vi "Aging Control Panel.vi"() -> ()   [LabVIEW 2020]
uses:
  typedefs/LED Controller Messages.ctl
  typedefs/TEC Queue Messages.ctl
  <vilib>/Utility/file.llb/Read Delimited Spreadsheet (string).vi
  Aging Control Panel_WT-v2 Backup/EC-Lab Development Package/Examples/Labview/V12/StartStopPause.vi
  Aging Control Panel_WT-v2 Backup/EC-Lab Development Package/Examples/Labview/V12/IntensityTemperature.vi
  <vilib>/Utility/file.llb/Write Delimited Spreadsheet (DBL).vi
panel:
  out "ControlTable2":dbl[][](array[numeric])
  out "Automatic Control Active H2":bool
  out "started last 2":timestamp
  out "TempArray":dbl[](array[numeric])=[29.1702938079834, 29.312671661376953, 29.52701187133789, 29.476533889770508, 31.52231216430664, 31.57969856262207, 31.603687286376953, 31.590633392333984]
  out "ControlTable1":dbl[][](array[numeric])
  out "started last":timestamp
  out "stopped":bool=TRUE
  out "Automatic Control Active H1":bool
  out "COM Done":bool
  out "Auto Done":bool
  out "TEC Done":bool
  out "index":i32
  in  "Tab Control":T1(tab)=enum."MagicControl"
  in  "ALL TEC SET A":bool caption="Light Off A"
  in  "cell A set":dbl=25.0
  in  "ALL TEC OFF B":bool caption="Light Off A"
  in  "ALL TEC ON B":bool caption="Light Off A"
  in  "ALL TEC OFF A":bool caption="Light Off A"
  in  "ALL TEC ON A":bool caption="Light Off A"
  in  "cell 1A set":dbl=25.0
  in  "cell 2A set":dbl=25.0
  in  "cell 3A set":dbl=25.0
  in  "cell 4A set":dbl=25.0
  out "cell 4A actual":dbl=29.476533889770508
  out "cell 3A actual":dbl=29.52701187133789
  out "cell 2A actual":dbl=29.312671661376953
  out "cell 1A actual":dbl=29.1702938079834
  out "Light Level B":dbl=-0.001053811659192825 caption="Light Level" format="%#_3g"
  out "Light Level A":dbl=-0.0009170305676855891 caption="Light Level" format="%#_3g"
  in  "cell 1B set":dbl=25.0
  in  "cell 2B set":dbl=25.0
  in  "cell 3B set":dbl=25.0
  in  "cell 4B set":dbl=25.0
  out "cell 4B actual":dbl=31.590633392333984
  out "cell 3B actual":dbl=31.603687286376953
  out "cell 2B actual":dbl=31.57969856262207
  out "cell 1B actual":dbl=31.52231216430664
  in  "Light Level set A":dbl(slide)=-1.0 scale=1e-05..10.0
  in  "Light Off A":bool
  in  "Light 1sun A":bool caption="Light Off A"
  in  "Light 0.1sun A":bool caption="Light Off A"
  in  "Light 0.01sun A":bool caption="Light Off A"
  in  "Light 1e-3sun A":bool caption="Light Off A"
  in  "Light 1e-4sun A":bool caption="Light Off A"
  in  "cell 1A ena":bool caption="enable"
  in  "cell 2A ena":bool caption="enable"
  in  "cell 3A ena":bool caption="enable"
  in  "cell 4A ena":bool caption="enable"
  in  "cell 1B ena":bool caption="enable"
  in  "cell 2B ena":bool caption="enable"
  in  "cell 3B ena":bool caption="enable"
  in  "cell 4B ena":bool caption="enable"
  out "TEC 1A Status":bool
  out "TEC 4A Status":bool
  out "TEC 3A Status":bool
  out "TEC 2A Status":bool
  out "TEC 4B Status":bool
  out "TEC 1B Status":bool
  out "TEC 3B Status":bool
  out "TEC 2B Status":bool
  in  "Light Level set B":dbl(slide)=-1.0 scale=1e-05..10.0
  in  "Light 1e-4sun B":bool caption="Light Off A"
  in  "Light 1e-3sun B":bool caption="Light Off A"
  in  "Light 0.01sun B":bool caption="Light Off A"
  in  "Light 0.1sun B":bool caption="Light Off A"
  in  "Light 1sun B":bool caption="Light Off A"
  in  "Light Off B":bool caption="Light Off A"
  in  "cell B set":dbl=25.0
  in  "ALL TEC SET B":bool caption="Light Off A"
  in  "Light Range A":bool=TRUE
  in  "Light Range B":bool=TRUE
  out "Temperature Monitor B":dbl[][](graph)=[[31.52231216430664, 31.57969856262207, 31.603687286376953, 31.590633392333984]]
  out "Temperature Monitor A":dbl[][](graph)=[[29.1702938079834, 29.312671661376953, 29.52701187133789, 29.476533889770508]]
  out "Light Level Monitor A":dbl(graph)=-0.0009170305676855891 caption="Cell A"
  out "Light Level Monitor B":dbl(graph)=-0.001053811659192825 caption="Cell B"
  in  "LED Auto-Connect":bool caption="Auto-Connect"
  in  "LED Disconnect":bool
  in  "LED Connect":bool
  in  "Dynamic Offset Cor.":bool=TRUE
  in  "TEC Reset":bool[](array[boolean])=[FALSE, FALSE, FALSE, FALSE, FALSE, FALSE, FALSE, FALSE] caption="Reset"
  in  "Regulation Mode A":bool=TRUE
  in  "LED Controller COM Port":refnum<visa-resource-name>="COM3"
  out "LED Controller Status":bool caption="Status"
  in  "High Light 1 Sun Level A":dbl=458.0 caption="1 Sun Level"
  in  "Low Light 1 Sun Level A":dbl=45800.0 caption="Low Light"
  in  "Light level raw A":dbl=-457.42
  in  "TEC COM Ports":refnum<visa-resource-name>[](array[refnum])=["COM6", "COM11", "COM10", "COM9", "COM4", "COM8", "COM5", "COM7"]
  out "TEC COM Status":bool[](array[boolean]) caption="Status"
  in  "TEC Auto-Detect":bool
  in  "TEC Connect":bool
  in  "TEC Disconnect":bool
  in  "TEC Address":u16(ring)=8 items=["ALL", "TEC 1A", "TEC 2A", "TEC 3A", "TEC 4A", "TEC 1B", "TEC 2B", "TEC 3B", "TEC 4B"]
  out "Diode Raw A":dbl=-1.0 format="%#_4g"
  out "Diode Raw B":dbl=-0.1 format="%#_4g"
  in  "Light level raw B":dbl=-445.97
  in  "Low Light 1 Sun Level B":dbl=44600.0 caption="Low Light"
  in  "High Light 1 Sun Level B":dbl=446.0 caption="High Light"
  in  "Regulation Mode B":bool
  out "TEC Voltage":dbl[](array[numeric])=[0.011975087225437164, 0.014526362530887127, 0.01483153272420168, 0.016552748158574104, 0.019128425046801567, 0.013830574229359627, 0.012988276779651642, 0.016076650470495224] caption="Voltage" format="%#.4g"
  out "TEC Current":dbl[](array[numeric])=[-0.0009887698106467724, -0.0016967777628451586, -0.0005615238915197551, -0.004669190384447575, -0.004687500651925802, -0.0027221685741096735, -0.0019592291209846735, -0.004602051340043545] caption="Current" format="%#.4g"
  in  "High Light Offset A":dbl=-0.5800000000000002 caption="Offset"
  in  "Low Light Offset A":dbl=-0.5100000000000001 caption="Low Light"
  in  "High Light Offset B":dbl=-0.03 caption="Offset"
  in  "Low Light Offset B":dbl=0.11999999999999998
  out "LED Driver Ground Offset (mV)":dbl=0.4
  in  "TEC Auto-Connect":bool caption="Auto-Connect"
  in  "TEC monitor\nperiod (ms)":i32=500
  in  "LED monitor\nperiod (ms)":i32=500
  in  "LED Slide reactivity (ms)":i32=250
  in  "TimingList2":i32(listbox)=-1
  out "Active Row 2":i32 caption="Active Row"
  out "started at 2":timestamp caption="started at"
  in  "RemoveRow1":bool caption="Light Off A"
  in  "AddRow1":bool caption="Light Off A"
  in  "SaveControlTable":bool caption="Light Off A"
  in  "LoadControlTable":bool caption="Light Off A"
  in  "TimingList1":i32(listbox)=-1
  in  "StartMagicControl":bool caption="Light Off A"
  in  "StopMagicControl":bool caption="Light Off A"
  out "started at":timestamp
  out "ElapsedTime":dbl
  out "Active Row":i32
  out "Current Row":dbl
  in  "loop to row":i32
  in  "loop to row 2":i32 caption="loop to row"
  out "Current Row 2":dbl caption="Current Row"
  out "ElapsedTime 2":dbl caption="ElapsedTime"
  in  "LoadControlTable 2":bool caption="Light Off A"
  in  "SaveControlTable 2":bool caption="Light Off A"
  in  "AddRow2":bool caption="Light Off A"
  in  "RemoveRow2":bool caption="Light Off A"
  in  "StartMagicControl 2":bool caption="Light Off A"
  in  "StopMagicControl 2":bool caption="Light Off A"
  out "StartStopPauseArray1":bool[][](array[boolean]) caption="Holder 1\nStart Stop Pause"
  out "StartStopPauseArray2":bool[][](array[boolean]) caption="Holder 2\nStart Stop Pause"
  in  "stop":bool
  # "3A"
  # "4B"
  # "3B"
  # "4A"
  # "1B"
  # "2A"
  # "1A"
  # "2B"
  # "LED A"
  # "LED B"
  # "1 Sun Level"
  # "High Light"
  # "Active (light green, on) entries will overwrite the commands in the AgingControl.\nNon-active entries will not do anything."
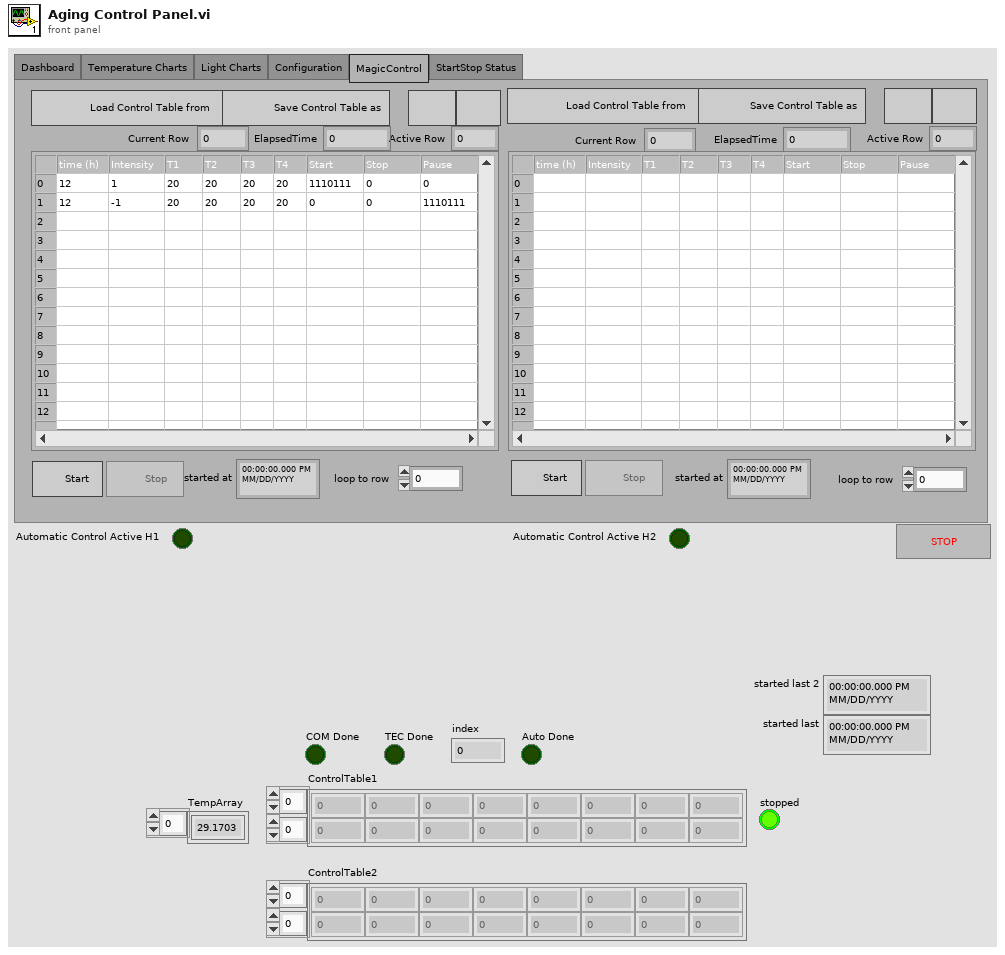
[diagram p1: front panel]
types:
  T1 = enum32{"Dashboard", "Temperature Charts", "Light Charts", "Configuration", "MagicControl", "StartStop Status"}
  T2 = cluster{"A Current":bool, "B Current":bool, "A lastupdate":u32, "B lastupdate":u32, "SetRange A":bool, "SetRange B":bool}
  T3 = cluster{"MODE A":bool, "MODE B":bool, "RANGE A":bool, "RANGE B":bool}
  T4 = typedef "TEC Queue Messages.ctl" = enum16{"Auto Detect", "Connect", "Disconnect", "Exit", "Set Temp", "Output Ena", "RESET"}
  T5 = typedef "LED Controller Messages.ctl" = enum16{"Connect", "Disconnect", "Exit", "Set Mode A", "Set Mode B", "Set Range A", "Set Range B", "Set Output A", "Set Output B"}
  T6 = enum8{"Enabled", "Disabled", "Disabled and Grayed Out"}
  T7 = cluster{"LED Controller COM Port":refnum<visa-resource-name>, i32}
  T8 = cluster{"LED Controller COM Port":refnum<visa-resource-name>, "TEC ID":i32}
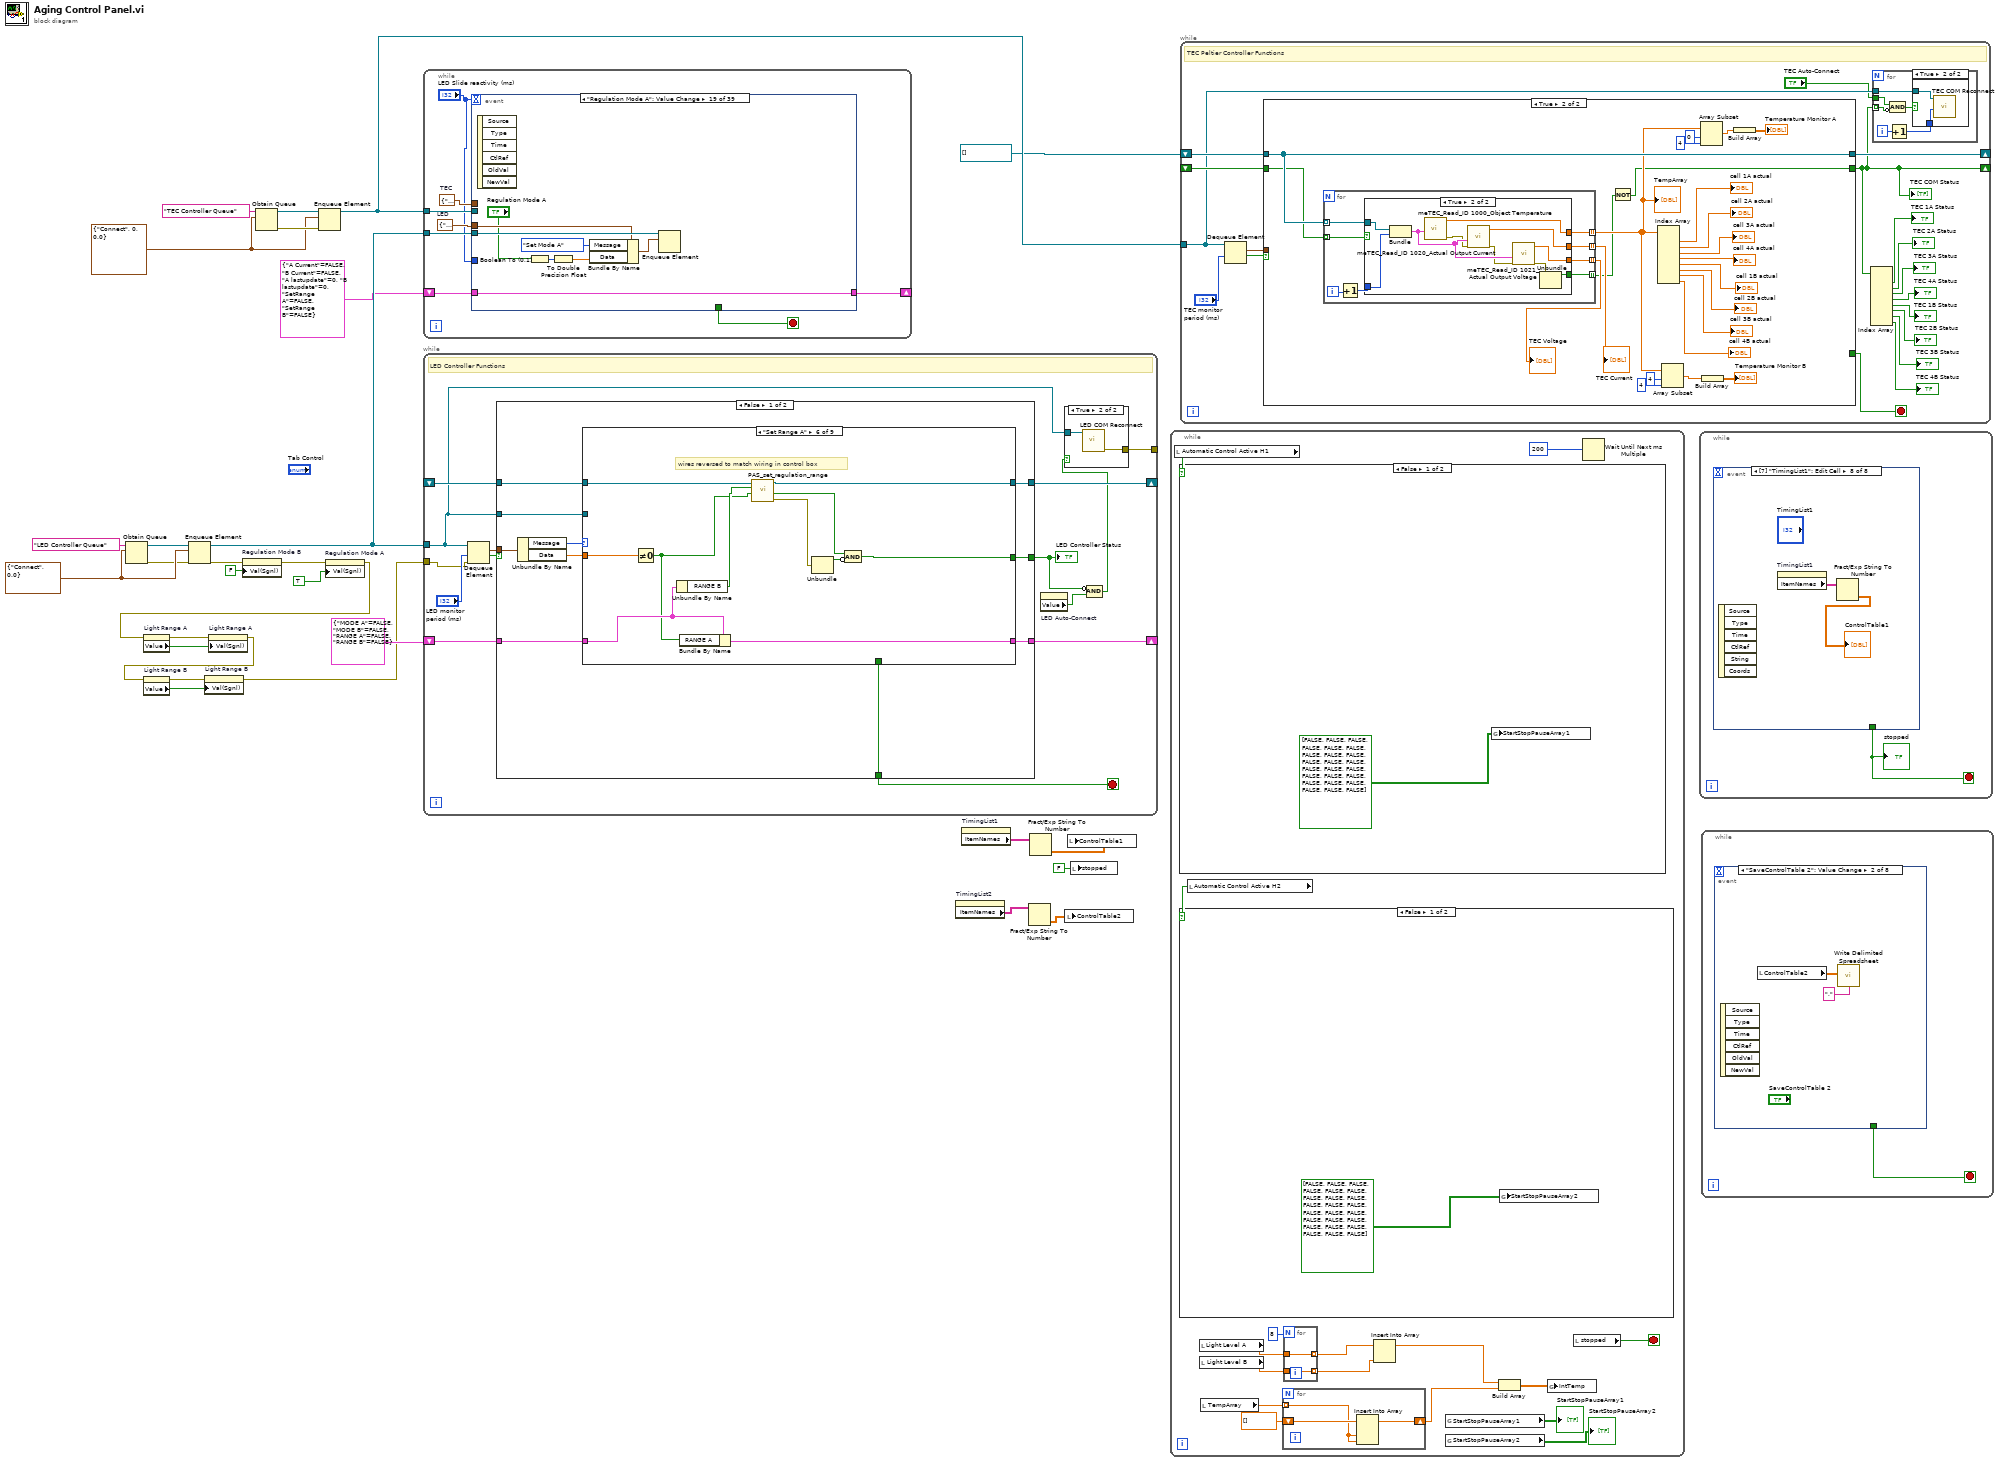
[diagram p0: block diagram]
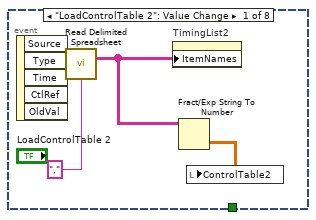
[diagram p2: hidden frame]
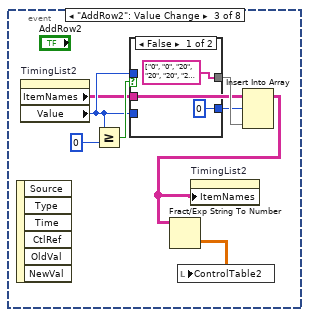
[diagram p3: hidden frame]
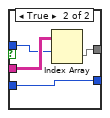
[diagram p4: hidden frame]
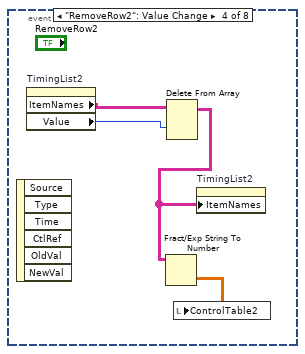
[diagram p5: hidden frame]
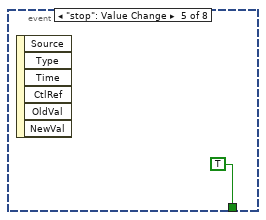
[diagram p6: hidden frame]
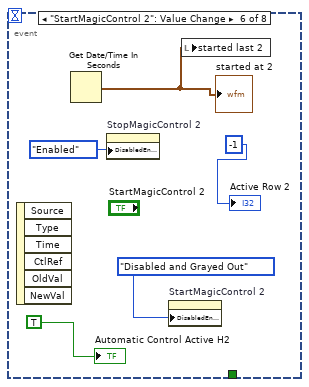
[diagram p7: hidden frame]
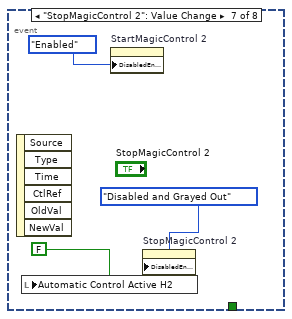
[diagram p8: hidden frame]
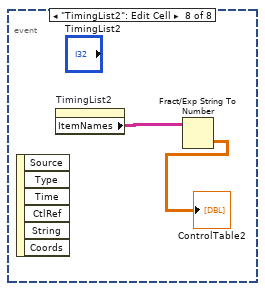
[diagram p9: hidden frame]
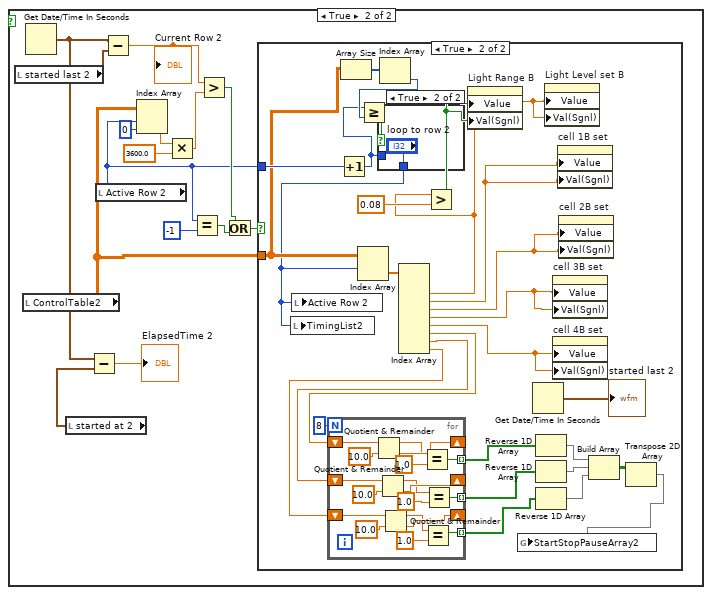
[diagram p10: hidden frame]
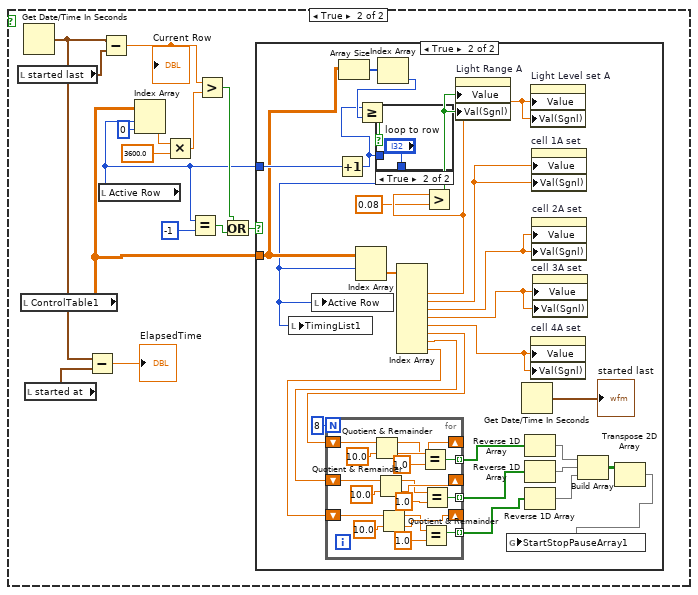
[diagram p13: hidden frame]
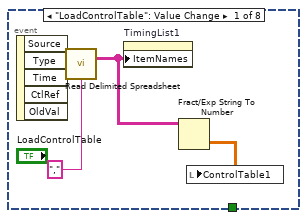
[diagram p16: hidden frame]
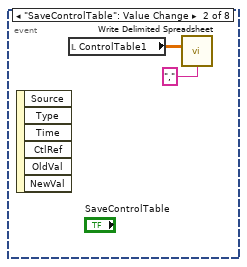
[diagram p17: hidden frame]
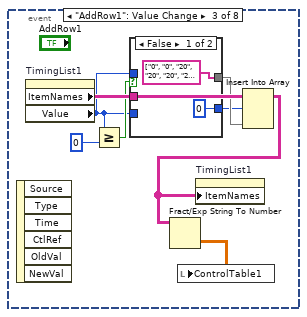
[diagram p18: hidden frame]
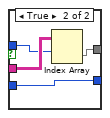
[diagram p19: hidden frame]
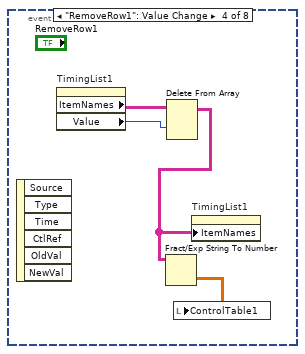
[diagram p20: hidden frame]
diagram:
  w24 = cluster{"Message":T4, "TEC ID":i32, "Data":dbl} {"Message"=enum."Connect", "TEC ID"=0, "Data"=0.0}
  w27 = cluster{"Message":T5, "Data":dbl} {"Message"=enum."Connect", "Data"=0.0}
  n1 = Obtain Queue(name (unnamed)="LED Controller Queue", element data type=w27) -> (queue out=w28:refnum<queue>, error out=w26:errorcluster)  [unwired: 3 in, 1 out]
  n2 = Enqueue Element(queue=w28, element=w27, error in (no error)=w26) -> (queue out=w17:refnum<queue>, error out=w18:errorcluster)  [unwired: 1 in, 1 out]
  n3 = property on="Regulation Mode B" class="Bool (strict)"(error in=w18, "Val(Sgnl)"=FALSE ("Value (Signaling)")) -> (error out=w16:errorcluster)  [unwired: 1 in, 1 out]
  n4 = Obtain Queue(name (unnamed)="TEC Controller Queue", element data type=w24) -> (queue out=w23:refnum<queue>, error out=w25:errorcluster)  [unwired: 3 in, 1 out]
  n5 = Enqueue Element(queue=w23, element=w24, error in (no error)=w25) -> (queue out=w21:refnum<queue>)  [unwired: 1 in, 2 out]
  n6 = property on="Regulation Mode A" class="Bool (strict)"(error in=w16, "Val(Sgnl)"=TRUE ("Value (Signaling)")) -> (error out=w9:errorcluster)  [unwired: 1 in, 1 out]
  n7 = property on="Light Range A" class="Bool (strict)"(error in=w9) -> (error out=w12:errorcluster, "Value"=w13:bool)  [unwired: 1 in, 1 out]
  n8 = property on="Light Range A" class="Bool (strict)"(error in=w12, "Val(Sgnl)"=w13) -> (error out=w8:errorcluster)  [unwired: 1 in, 1 out]
  n9 = property on="Light Range B" class="Bool (strict)"(error in=w8) -> (error out=w10:errorcluster, "Value"=w11:bool)  [unwired: 1 in, 1 out]
  n10 = property on="Light Range B" class="Bool (strict)"(error in=w10, "Val(Sgnl)"=w11) -> (error out=w7:errorcluster)  [unwired: 1 in, 1 out]
  n11 = while {
    tunnel: w17 -> [w36]
    tunnel: w21 -> [w34]
    shift-right: [w31] -> _
    shift-left: T2 {"A Current"=FALSE, "B Current"=FALSE, "A lastupdate"=0, "B lastupdate"=0, "SetRange A"=FALSE, "SetRange B"=FALSE} -> [w32]
    stop <- w37 stop-if-true
    w33 = cluster{"Message":T4, "TEC ID":i32, "Data":dbl} {"Message"=enum."Connect", "TEC ID"=0, "Data"=0.0}  # TEC
    w35 = cluster{"Message":T5, "Data":dbl} {"Message"=enum."Set Output B", "Data"=0.0}  # LED
    n12 = event shown="[18] \"Regulation Mode A\": Value Change" {
      selector: _ -> [_ _ _ _ _ _ _ _ _ _ _ _ _ _ _ _ _ _ _ _ _ _ _ _ _ _ _ _ _ _ _ _ _ _ _ _ _ _ _]
      dyn-events: _ -> [_ _ _ _ _ _ _ _ _ _ _ _ _ _ _ _ _ _ _ _ _ _ _ _ _ _ _ _ _ _ _ _ _ _ _ _ _ _ _]
      timeout: "LED Slide reactivity (ms)" -> [_ _ _ _ _ _ _ _ _ _ _ _ _ _ _ _ _ _ _ _ _ _ _ _ _ _ _ _ _ _ _ _ _ _ _ _ _ _ _]
      tunnel: [_ TRUE _ _ _ _ _ _ _ _ _ _ _ _ _ _ _ _ _ _ _ _ _ _ _ _ _ _ _ _ _ _ _ _ _ _ _ _ _] -> w37
      tunnel: w36 -> [_ w66 _ _ _ _ _ _ _ _ _ _ _ _ _ _ w152 w170 w191 w199 w207 w236 _ _ _ _ _ _ _ _ _ _ _ _ _ w379 w386 _ w428]
      tunnel: w35 -> [_ w58 _ _ _ _ _ _ _ _ _ _ _ _ _ _ w151 w169 w190 w198 w204 w233 _ _ _ _ _ _ _ _ _ _ _ _ _ w381 w385 _ w430]
      tunnel: w34 -> [_ w69 _ _ _ _ _ _ _ _ _ _ _ _ _ _ _ _ _ _ _ _ w264 w277 _ _ _ _ _ _ w326 _ w357 w366 w375 _ _ w407 _]
      tunnel: w33 -> [_ w64 _ _ _ _ _ _ _ _ _ _ _ _ _ _ _ _ _ _ _ _ w263 w276 _ _ _ _ _ _ w325 _ w356 w365 w374 _ _ w406 _]
      tunnel: w32 -> [w42 w56 w75 w101 w124 w126 w128 w130 w132 w134 w136 w138 w140 w142 w144 w146 w149 w168 w184 w192 w202 w231 w256 w266 w278 w286 w294 w302 w310 w315 w320 w329 w350 w358 w367 w376 w384 w405 w425]
      tunnel: [w38 w56 w74 w99 w124 w126 w128 w130 w132 w134 w136 w138 w140 w142 w144 w146 w148 w167 w184 w192 w201 w230 w256 w266 w278 w286 w294 w302 w310 w315 w320 w329 w350 w358 w367 w376 w384 w405 w425] -> w31
      tunnel: "LED Slide reactivity (ms)" -> [_ _ w72 w98 _ _ _ _ _ _ _ _ _ _ _ _ _ _ _ _ _ _ _ _ _ _ _ _ _ _ _ _ _ _ _ _ _ _ _]
      event Timeout {
        n13 = event-data() -> ("Time"=w40:u32)  [unwired: 1 in, 2 out]
        n14 = Unbundle By Name(w42) -> ("A Current"=w43:bool, "B Current"=w39:bool)
        n15 = case shown="False" w43 {
          tunnel: w42 -> [w53 w55]
          tunnel: w40 -> [w52 _]
          tunnel: [w50 w55] -> w41
          frame False {
            n16 = property on="Light level raw A" class="DigNum (strict)"() -> ("Value"=w54:dbl)  [unwired: 2 in, 2 out]
            n17 = Bundle By Name(cluster=w53, "A Current"=TRUE, "A lastupdate"=w52) -> (w50:T2)
            n18 = property on="Light level raw A" class="DigNum (strict)"("Val(Sgnl)"=w54) -> ()  [unwired: 2 in, 2 out]
          }
          frame True {
          }
        }
        n19 = case shown="False" w39 {
          tunnel: w41 -> [w47 w49]
          tunnel: w40 -> [w46 _]
          tunnel: [w44 w49] -> w38
          frame False {
            n20 = property on="Light level raw B" class="DigNum (strict)"() -> ("Value"=w48:dbl)  [unwired: 2 in, 2 out]
            n21 = Bundle By Name(cluster=w47, "B Current"=TRUE ("A Current"), "B lastupdate"=w46) -> (w44:T2)
            n22 = property on="Light level raw B" class="DigNum (strict)"("Val(Sgnl)"=w48) -> ()  [unwired: 2 in, 2 out]
          }
          frame True {
          }
        }
      }
      event "stop": Value Change {
        n23 = event-data() -> ()  [unwired: 1 in, 6 out]
        n24 = Bundle By Name(cluster=w58, "Message"=LED_Controller_Messages."Disconnect") -> (w59:cluster{"Message":T5, "Data":dbl})
        n25 = Bundle By Name(cluster=w58, "Message"=LED_Controller_Messages."Exit") -> (w57:cluster{"Message":T5, "Data":dbl})
        n26 = Bundle By Name(cluster=w64, "Message"=TEC_Queue_Messages."Disconnect") -> (w67:cluster{"Message":T4, "TEC ID":i32, "Data":dbl})
        n27 = Bundle By Name(cluster=w64, "Message"=TEC_Queue_Messages."Exit") -> (w62:cluster{"Message":T4, "TEC ID":i32, "Data":dbl})
        n28 = Enqueue Element(queue=w66, element=w59) -> (queue out=w61:refnum<queue>)  [unwired: 2 in, 2 out]
        n29 = Enqueue Element(queue=w69, element=w67) -> (queue out=w63:refnum<queue>)  [unwired: 2 in, 2 out]
        n30 = Enqueue Element(queue=w61, element=w57) -> ()  [unwired: 2 in, 3 out]
        n31 = Enqueue Element(queue=w63, element=w62) -> ()  [unwired: 2 in, 3 out]
      }
      event "Light Level set B": Value Change {
        n32 = event-data() -> ("Time"=w73:u32)  [unwired: 1 in, 5 out]
        n33 = Unbundle By Name(w75) -> ("B lastupdate"=w78:u32)
        n34 = property on="Light Range B" class="Bool (strict)"() -> ("Value"=w82:bool)  [unwired: 2 in, 2 out]
        n35 = Subtract(x=w73, y=w78) -> (x-y=w77:u32)
        n36 = Select(t="High Light 1 Sun Level B", s=w82, f="Low Light 1 Sun Level B") -> (s? t:f=w87:dbl)
        n37 = Greater?(x=w77, y=w72) -> (0:w76:bool)
        n38 = Multiply(x=w87, y="Light Level set B") -> (x*y=w81:dbl)
        n39 = Select(t="High Light Offset B", s=w82, f="Low Light Offset B") -> (s? t:f=w79:dbl)
        n40 = Subtract(x=w81, y=w79) -> (x-y=w80:dbl)
        n41 = case shown="True" w76 {
          selector: w76 -> [w90 w93]
          tunnel: w80 -> [w89 w97]
          tunnel: w75 -> [w92 w96]
          tunnel: [w91 w95] -> w74
          tunnel: w73 -> [_ w94]
          frame False {
            n42 = Bundle By Name(cluster=w92, "B Current"=w90) -> (w91:T2)
            n43 = property on="Light level raw B" class="DigNum (strict)"("Value"=w89) -> ()  [unwired: 2 in, 2 out]
          }
          frame True {
            n44 = Bundle By Name(cluster=w96, "B Current"=w93, "B lastupdate"=w94) -> (w95:T2)
            n45 = property on="Light level raw B" class="DigNum (strict)"("Val(Sgnl)"=w97) -> ()  [unwired: 2 in, 2 out]
          }
        }
      }
      event "Light Level set A": Value Change {
        n46 = event-data() -> ("Time"=w100:u32)  [unwired: 1 in, 5 out]
        n47 = Unbundle By Name(w101) -> ("A lastupdate"=w104:u32)
        n48 = property on="Light Range A" class="Bool (strict)"() -> ("Value"=w108:bool)  [unwired: 2 in, 2 out]
        n49 = Subtract(x=w100, y=w104) -> (x-y=w103:u32)
        n50 = Select(t="High Light 1 Sun Level A", s=w108, f="Low Light 1 Sun Level A") -> (s? t:f=w113:dbl)
        n51 = Greater?(x=w103, y=w98) -> (0:w102:bool)
        n52 = Multiply(x=w113, y="Light Level set A") -> (x*y=w107:dbl)
        n53 = Select(t="High Light Offset A", s=w108, f="Low Light Offset A") -> (s? t:f=w105:dbl)
        n54 = Subtract(x=w107, y=w105) -> (x-y=w106:dbl)
        n55 = case shown="False" w102 {
          selector: w102 -> [w117 w121]
          tunnel: w106 -> [w115 w123]
          tunnel: w101 -> [w118 w122]
          tunnel: w100 -> [_ w120]
          tunnel: [w116 w119] -> w99
          frame False {
            n56 = Bundle By Name(cluster=w118, "A Current"=w117) -> (w116:T2)
            n57 = property on="Light level raw A" class="DigNum (strict)"("Value"=w115) -> ()  [unwired: 2 in, 2 out]
          }
          frame True {
            n58 = Bundle By Name(cluster=w122, "A Current"=w121, "A lastupdate"=w120) -> (w119:T2)
            n59 = property on="Light level raw A" class="DigNum (strict)"("Val(Sgnl)"=w123) -> ()  [unwired: 2 in, 2 out]
          }
        }
      }
      event "Light 1sun B": Value Change {
        n60 = event-data() -> ()  [unwired: 1 in, 6 out]
        n61 = property on="Light Level set B" class="Slide (strict)"("Val(Sgnl)"=1.0 ("Value (Signaling)")) -> ()  [unwired: 2 in, 2 out]
      }
      event "Light 1sun A": Value Change {
        n62 = event-data() -> ()  [unwired: 1 in, 6 out]
        n63 = property on="Light Level set A" class="Slide (strict)"("Val(Sgnl)"=1.0 ("Value (Signaling)")) -> ()  [unwired: 2 in, 2 out]
      }
      event "Light 0.1sun B": Value Change {
        n64 = event-data() -> ()  [unwired: 1 in, 6 out]
        n65 = property on="Light Level set B" class="Slide (strict)"("Val(Sgnl)"=0.1 ("Value (Signaling)")) -> ()  [unwired: 2 in, 2 out]
      }
      event "Light 0.1sun A": Value Change {
        n66 = event-data() -> ()  [unwired: 1 in, 6 out]
        n67 = property on="Light Level set A" class="Slide (strict)"("Val(Sgnl)"=0.1 ("Value (Signaling)")) -> ()  [unwired: 2 in, 2 out]
      }
      event "Light 0.01sun B": Value Change {
        n68 = event-data() -> ()  [unwired: 1 in, 6 out]
        n69 = property on="Light Level set B" class="Slide (strict)"("Val(Sgnl)"=0.01 ("Value (Signaling)")) -> ()  [unwired: 2 in, 2 out]
      }
      event "Light 0.01sun A": Value Change {
        n70 = event-data() -> ()  [unwired: 1 in, 6 out]
        n71 = property on="Light Level set A" class="Slide (strict)"("Val(Sgnl)"=0.01 ("Value (Signaling)")) -> ()  [unwired: 2 in, 2 out]
      }
      event "Light 1e-3sun B": Value Change {
        n72 = event-data() -> ()  [unwired: 1 in, 6 out]
        n73 = property on="Light Level set B" class="Slide (strict)"("Val(Sgnl)"=0.001 ("Value (Signaling)")) -> ()  [unwired: 2 in, 2 out]
      }
      event "Light 1e-3sun A": Value Change {
        n74 = event-data() -> ()  [unwired: 1 in, 6 out]
        n75 = property on="Light Level set A" class="Slide (strict)"("Val(Sgnl)"=0.001 ("Value (Signaling)")) -> ()  [unwired: 2 in, 2 out]
      }
      event "Light 1e-4sun B": Value Change {
        n76 = event-data() -> ()  [unwired: 1 in, 6 out]
        n77 = property on="Light Level set B" class="Slide (strict)"("Val(Sgnl)"=0.0001 ("Value (Signaling)")) -> ()  [unwired: 2 in, 2 out]
      }
      event "Light 1e-4sun A": Value Change {
        n78 = event-data() -> ()  [unwired: 1 in, 6 out]
        n79 = property on="Light Level set A" class="Slide (strict)"("Val(Sgnl)"=0.0001 ("Value (Signaling)")) -> ()  [unwired: 2 in, 2 out]
      }
      event "Light Off B": Value Change {
        n80 = event-data() -> ()  [unwired: 1 in, 6 out]
        n81 = property on="Light Level set B" class="Slide (strict)"("Val(Sgnl)"=-1.0 ("Value (Signaling)")) -> ()  [unwired: 2 in, 2 out]
      }
      event "Light Off A": Value Change {
        n82 = event-data() -> ()  [unwired: 1 in, 6 out]
        n83 = property on="Light Level set A" class="Slide (strict)"("Val(Sgnl)"=-1.0 ("Value (Signaling)")) -> ()  [unwired: 2 in, 2 out]
      }
      event "Light Range B": Value Change {
        n84 = event-data() -> ()  [unwired: 1 in, 6 out]
        n85 = property on="Light Level set B" class="Slide (strict)"() -> (error out=w153:errorcluster, "Value"=w154:dbl)  [unwired: 2 in, 1 out]
        n86 = case shown="False" "Light Range B" {
          selector: "Light Range B" -> [w156 _]
          tunnel: w152 -> [w162 _]
          tunnel: w151 -> [w161 _]
          tunnel: w149 -> [w155 w165]
          tunnel: [w155 w164] -> w148
          frame False {
            n87 = Boolean To (0,1)(Boolean=w156) -> (0, 1=w159:i16)
            n88 = To Double Precision Float(number=w159) -> (double precision float=w158:dbl)
            n89 = Bundle By Name(cluster=w161, "Message"=LED_Controller_Messages."Set Range B", "Data"=w158) -> (w157:cluster{"Message":T5, "Data":dbl})
            n90 = Enqueue Element(queue=w162, element=w157) -> ()  [unwired: 2 in, 3 out]
          }
          frame True {
            n91 = Bundle By Name(cluster=w165, "SetRange B"=TRUE) -> (w164:T2)
          }
        }
        n92 = property on="Light Level set B" class="Slide (strict)"(error in=w153, "Val(Sgnl)"=w154) -> ()  [unwired: 1 in, 2 out]
      }
      event "Light Range A": Value Change {
        n93 = event-data() -> ()  [unwired: 1 in, 6 out]
        n94 = property on="Light Level set A" class="Slide (strict)"() -> (error out=w171:errorcluster, "Value"=w172:dbl)  [unwired: 2 in, 1 out]
        n95 = case shown="True" "Light Range A" {
          selector: "Light Range A" -> [w174 _]
          tunnel: w170 -> [w180 _]
          tunnel: w169 -> [w179 _]
          tunnel: w168 -> [w173 w183]
          tunnel: [w173 w182] -> w167
          frame False {
            n96 = Boolean To (0,1)(Boolean=w174) -> (0, 1=w177:i16)
            n97 = To Double Precision Float(number=w177) -> (double precision float=w176:dbl)
            n98 = Bundle By Name(cluster=w179, "Message"=LED_Controller_Messages."Set Range A", "Data"=w176) -> (w175:cluster{"Message":T5, "Data":dbl})
            n99 = Enqueue Element(queue=w180, element=w175) -> ()  [unwired: 2 in, 3 out]
          }
          frame True {
            n100 = Bundle By Name(cluster=w183, "SetRange A"=TRUE ("SetRange B")) -> (w182:T2)
          }
        }
        n101 = property on="Light Level set A" class="Slide (strict)"(error in=w171, "Val(Sgnl)"=w172) -> ()  [unwired: 1 in, 2 out]
      }
      event "Regulation Mode A": Value Change {
        n102 = event-data() -> ()  [unwired: 1 in, 6 out]
        n103 = Boolean To (0,1)(Boolean="Regulation Mode A") -> (0, 1=w188:i16)
        n104 = To Double Precision Float(number=w188) -> (double precision float=w187:dbl)
        n105 = Bundle By Name(cluster=w190, "Message"=LED_Controller_Messages."Set Mode A", "Data"=w187) -> (w186:cluster{"Message":T5, "Data":dbl})
        n106 = Enqueue Element(queue=w191, element=w186) -> ()  [unwired: 2 in, 3 out]
      }
      event "Regulation Mode B": Value Change {
        n107 = event-data() -> ()  [unwired: 1 in, 6 out]
        n108 = Boolean To (0,1)(Boolean="Regulation Mode B") -> (0, 1=w196:i16)
        n109 = To Double Precision Float(number=w196) -> (double precision float=w195:dbl)
        n110 = Bundle By Name(cluster=w198, "Message"=LED_Controller_Messages."Set Mode B", "Data"=w195) -> (w194:cluster{"Message":T5, "Data":dbl})
        n111 = Enqueue Element(queue=w199, element=w194) -> ()  [unwired: 2 in, 3 out]
      }
      event "Light level raw B": Value Change {
        n112 = event-data() -> ()  [unwired: 1 in, 6 out]
        n113 = Unbundle By Name(w202) -> ("SetRange B"=w203:bool)
        n114 = In Range and Coerce(upper limit=4900.0, x="Light level raw B", lower limit=-3.0) -> (coerced(x)=w206:dbl)  [unwired: 1 out]
        n115 = Bundle By Name(cluster=w204, "Message"=LED_Controller_Messages."Set Output B", "Data"=w206) -> (w211:cluster{"Message":T5, "Data":dbl})
        n116 = Enqueue Element(queue=w207, element=w211) -> (queue out=w205:refnum<queue>, error out=w200:errorcluster)  [unwired: 2 in, 1 out]
        n117 = case shown="True" w203 {
          selector: w203 -> [_ w216]
          tunnel: w205 -> [_ w225]
          tunnel: w204 -> [_ w224]
          tunnel: w202 -> [w213 w219]
          tunnel: [w213 w217] -> w201
          tunnel: w200 -> [_ w215]
          frame False {
          }
          frame True {
            n118 = flat-sequence {
              tunnel: w215 -> [w226]
              tunnel: [w226] -> w214
              frame #0 {
                n119 = Wait (ms)(milliseconds to wait=u32 100) -> ()  [unwired: 1 out]
              }
            }
            n120 = Boolean To (0,1)(Boolean=w216) -> (0, 1=w222:i16)
            n121 = Bundle By Name(cluster=w219, "SetRange B"=FALSE) -> (w217:T2)
            n122 = To Double Precision Float(number=w222) -> (double precision float=w221:dbl)
            n123 = Bundle By Name(cluster=w224, "Message"=LED_Controller_Messages."Set Range B", "Data"=w221) -> (w220:cluster{"Message":T5, "Data":dbl})
            n124 = Enqueue Element(queue=w225, element=w220, error in (no error)=w214) -> ()  [unwired: 1 in, 3 out]
          }
        }
      }
      event "Light level raw A": Value Change {
        n125 = event-data() -> ()  [unwired: 1 in, 6 out]
        n126 = Unbundle By Name(w231) -> ("SetRange A"=w232:bool)
        n127 = In Range and Coerce(upper limit=4900.0, x="Light level raw A", lower limit=-3.0) -> (coerced(x)=w235:dbl)  [unwired: 1 out]
        n128 = Bundle By Name(cluster=w233, "Message"=LED_Controller_Messages."Set Output A", "Data"=w235) -> (w239:cluster{"Message":T5, "Data":dbl})
        n129 = Enqueue Element(queue=w236, element=w239) -> (queue out=w234:refnum<queue>, error out=w229:errorcluster)  [unwired: 2 in, 1 out]
        n130 = case shown="True" w232 {
          selector: w232 -> [_ w244]
          tunnel: w234 -> [_ w253]
          tunnel: w233 -> [_ w252]
          tunnel: w231 -> [w241 w247]
          tunnel: [w241 w245] -> w230
          tunnel: w229 -> [_ w243]
          frame False {
          }
          frame True {
            n131 = flat-sequence {
              tunnel: w243 -> [w254]
              tunnel: [w254] -> w242
              frame #0 {
                n132 = Wait (ms)(milliseconds to wait=u32 100) -> ()  [unwired: 1 out]
              }
            }
            n133 = Boolean To (0,1)(Boolean=w244) -> (0, 1=w250:i16)
            n134 = Bundle By Name(cluster=w247, "SetRange A"=FALSE ("SetRange B")) -> (w245:T2)
            n135 = To Double Precision Float(number=w250) -> (double precision float=w249:dbl)
            n136 = Bundle By Name(cluster=w252, "Message"=LED_Controller_Messages."Set Range A", "Data"=w249) -> (w248:cluster{"Message":T5, "Data":dbl})
            n137 = Enqueue Element(queue=w253, element=w248, error in (no error)=w242) -> ()  [unwired: 1 in, 3 out]
          }
        }
      }
      event "cell 1A set", "cell 2A set", "cell 3A set", "cell 4A set", "cell 1B set", "cell 2B set", "cell 3B set", "cell 4B set": Value Change {
        n138 = event-data() -> ("CtlRef"=w265:refnum<vi>, "NewVal"=w260:dbl)  [unwired: 1 in, 4 out]
        n139 = To More Generic Class(target class=refnum<vi> refnum ("reference"), reference=w265) -> (generic class reference=w258:refnum<vi>)
        n140 = call "Extract Control Index.vi"("reference"=w258) -> ("index"=w261:i32)  [unwired: 10 in]
        n141 = Bundle By Name(cluster=w263, "Message"=TEC_Queue_Messages."Set Temp", "TEC ID"=w261, "Data"=w260) -> (w259:cluster{"Message":T4, "TEC ID":i32, "Data":dbl})
        n142 = Enqueue Element(queue=w264, element=w259) -> ()  [unwired: 2 in, 3 out]
      }
      event "cell 1A ena", "cell 2A ena", "cell 3A ena", "cell 4A ena", "cell 1B ena", "cell 2B ena", "cell 3B ena", "cell 4B ena": Value Change {
        n143 = event-data() -> ("CtlRef"=w269:refnum<vi>, "NewVal"=w273:bool)  [unwired: 1 in, 4 out]
        n144 = To More Generic Class(target class=refnum<vi> refnum ("reference"), reference=w269) -> (generic class reference=w268:refnum<vi>)
        n145 = Boolean To (0,1)(Boolean=w273) -> (0, 1=w271:i16)
        n146 = To Double Precision Float(number=w271) -> (double precision float=w270:dbl)
        n147 = call "Extract Control Index.vi"("reference"=w268) -> ("index"=w274:i32)  [unwired: 10 in]
        n148 = Bundle By Name(cluster=w276, "Message"=TEC_Queue_Messages."Output Ena", "TEC ID"=w274, "Data"=w270) -> (w272:cluster{"Message":T4, "TEC ID":i32, "Data":dbl})
        n149 = Enqueue Element(queue=w277, element=w272) -> ()  [unwired: 2 in, 3 out]
      }
      event "ALL TEC ON A": Value Change {
        n150 = event-data() -> ()  [unwired: 1 in, 6 out]
        n151 = property on="cell 1A ena" class="Bool (strict)"("Val(Sgnl)"=TRUE ("cell 1A ena")) -> (error out=w285:errorcluster)  [unwired: 2 in, 1 out]
        n152 = property on="cell 2A ena" class="Bool (strict)"(error in=w285, "Val(Sgnl)"=TRUE ("cell 2A ena")) -> (error out=w284:errorcluster)  [unwired: 1 in, 1 out]
        n153 = property on="cell 3A ena" class="Bool (strict)"(error in=w284, "Val(Sgnl)"=TRUE ("cell 3A ena")) -> (error out=w283:errorcluster)  [unwired: 1 in, 1 out]
        n154 = property on="cell 4A ena" class="Bool (strict)"(error in=w283, "Val(Sgnl)"=TRUE ("Value (Signaling)")) -> ()  [unwired: 1 in, 2 out]
      }
      event "ALL TEC OFF A": Value Change {
        n155 = event-data() -> ()  [unwired: 1 in, 6 out]
        n156 = property on="cell 1A ena" class="Bool (strict)"("Val(Sgnl)"=FALSE ("cell 1A ena")) -> (error out=w293:errorcluster)  [unwired: 2 in, 1 out]
        n157 = property on="cell 2A ena" class="Bool (strict)"(error in=w293, "Val(Sgnl)"=FALSE ("cell 2A ena")) -> (error out=w292:errorcluster)  [unwired: 1 in, 1 out]
        n158 = property on="cell 3A ena" class="Bool (strict)"(error in=w292, "Val(Sgnl)"=FALSE ("cell 3A ena")) -> (error out=w291:errorcluster)  [unwired: 1 in, 1 out]
        n159 = property on="cell 4A ena" class="Bool (strict)"(error in=w291, "Val(Sgnl)"=FALSE ("Value (Signaling)")) -> ()  [unwired: 1 in, 2 out]
      }
      event "ALL TEC ON B": Value Change {
        n160 = event-data() -> ()  [unwired: 1 in, 6 out]
        n161 = property on="cell 1B ena" class="Bool (strict)"("Val(Sgnl)"=TRUE ("cell 1A ena")) -> (error out=w301:errorcluster)  [unwired: 2 in, 1 out]
        n162 = property on="cell 2B ena" class="Bool (strict)"(error in=w301, "Val(Sgnl)"=TRUE ("cell 2A ena")) -> (error out=w300:errorcluster)  [unwired: 1 in, 1 out]
        n163 = property on="cell 3B ena" class="Bool (strict)"(error in=w300, "Val(Sgnl)"=TRUE ("cell 3A ena")) -> (error out=w299:errorcluster)  [unwired: 1 in, 1 out]
        n164 = property on="cell 4B ena" class="Bool (strict)"(error in=w299, "Val(Sgnl)"=TRUE ("Value (Signaling)")) -> ()  [unwired: 1 in, 2 out]
      }
      event "ALL TEC OFF B": Value Change {
        n165 = event-data() -> ()  [unwired: 1 in, 6 out]
        n166 = property on="cell 1B ena" class="Bool (strict)"("Val(Sgnl)"=FALSE ("cell 1A ena")) -> (error out=w309:errorcluster)  [unwired: 2 in, 1 out]
        n167 = property on="cell 2B ena" class="Bool (strict)"(error in=w309, "Val(Sgnl)"=FALSE ("cell 2A ena")) -> (error out=w308:errorcluster)  [unwired: 1 in, 1 out]
        n168 = property on="cell 3B ena" class="Bool (strict)"(error in=w308, "Val(Sgnl)"=FALSE ("cell 3A ena")) -> (error out=w307:errorcluster)  [unwired: 1 in, 1 out]
        n169 = property on="cell 4B ena" class="Bool (strict)"(error in=w307, "Val(Sgnl)"=FALSE ("Value (Signaling)")) -> ()  [unwired: 1 in, 2 out]
      }
      event "ALL TEC SET A": Value Change {
        n170 = event-data() -> ()  [unwired: 1 in, 6 out]
        n171 = property on="cell 1A set" class="DigNum (strict)"("Val(Sgnl)"="cell A set") -> (error out=w314:errorcluster)  [unwired: 2 in, 1 out]
        n172 = property on="cell 2A set" class="DigNum (strict)"(error in=w314, "Val(Sgnl)"="cell A set") -> (error out=w313:errorcluster)  [unwired: 1 in, 1 out]
        n173 = property on="cell 3A set" class="DigNum (strict)"(error in=w313, "Val(Sgnl)"="cell A set") -> (error out=w312:errorcluster)  [unwired: 1 in, 1 out]
        n174 = property on="cell 4A set" class="DigNum (strict)"(error in=w312, "Val(Sgnl)"="cell A set") -> ()  [unwired: 1 in, 2 out]
      }
      event "ALL TEC SET B": Value Change {
        n175 = event-data() -> ()  [unwired: 1 in, 6 out]
        n176 = property on="cell 1B set" class="DigNum (strict)"("Val(Sgnl)"="cell B set") -> (error out=w319:errorcluster)  [unwired: 2 in, 1 out]
        n177 = property on="cell 2B set" class="DigNum (strict)"(error in=w319, "Val(Sgnl)"="cell B set") -> (error out=w318:errorcluster)  [unwired: 1 in, 1 out]
        n178 = property on="cell 3B set" class="DigNum (strict)"(error in=w318, "Val(Sgnl)"="cell B set") -> (error out=w317:errorcluster)  [unwired: 1 in, 1 out]
        n179 = property on="cell 4B set" class="DigNum (strict)"(error in=w317, "Val(Sgnl)"="cell B set") -> ()  [unwired: 1 in, 2 out]
      }
      event "TEC Reset": Value Change {
        n180 = event-data() -> ()  [unwired: 1 in, 6 out]
        n181 = Search 1D Array(1D array="TEC Reset", element=TRUE) -> (index of element=w322:i32)  [unwired: 1 in]
        n182 = Increment(x=w322) -> (x+1=w321:i32)
        n183 = Bundle By Name(cluster=w325, "Message"=TEC_Queue_Messages."RESET", "TEC ID"=w321) -> (w327:cluster{"Message":T4, "TEC ID":i32, "Data":dbl})
        n184 = Enqueue Element(queue=w326, element=w327) -> ()  [unwired: 2 in, 3 out]
      }
      event "TEC Address": Value Change {
        n185 = event-data() -> ("NewVal"=w332:u16)  [unwired: 1 in, 5 out]
        n186 = property on="TEC COM Status" class="Arr (strict)"() -> ("Value"=w330:bool[])  [unwired: 2 in, 2 out]
        n187 = Not Equal To 0?(x=w332) -> (x != 0?=w331:bool)
        n188 = case shown="False" w331 {
          tunnel: w332 -> [_ w345]
          tunnel: w330 -> [w341 w343]
          frame False {
            w333 = T6."Enabled" ("Disabled")
            w334 = T6."Disabled and Grayed Out" ("Disabled")
            n189 = Boolean Array To Number(Boolean array=w341) -> (number=w340:u32)
            n190 = Equal To 0?(x=w340) -> (x = 0?=w336:bool)
            n191 = Equal?(x=w340, y=u32 255) -> (x = y?=w335:bool)
            n192 = Select(t=w334, s=w336, f=w333) -> (s? t:f=w338:T6)
            n193 = Select(t=w334, s=w335, f=w333) -> (s? t:f=w337:T6)
            n194 = property on="TEC Disconnect" class="Bool"("DisabledEnum"=w338) -> ()  [unwired: 2 in, 2 out]
            n195 = property on="TEC Connect" class="Bool"("DisabledEnum"=w337) -> ()  [unwired: 2 in, 2 out]
          }
          frame True {
            n196 = Decrement(x=w345) -> (x-1=w344:u16)
            n197 = Index Array(array=w343, index=w344) -> (element=w342:bool)
            n198 = case shown="True" w342 {
              frame False {
                n199 = property on="TEC Disconnect" class="Bool"("DisabledEnum"=T6."Disabled and Grayed Out" ("Disabled")) -> ()  [unwired: 2 in, 2 out]
                n200 = property on="TEC Connect" class="Bool"("DisabledEnum"=T6."Enabled" ("Disabled")) -> ()  [unwired: 2 in, 2 out]
              }
              frame True {
                n201 = property on="TEC Disconnect" class="Bool"("DisabledEnum"=T6."Enabled" ("Disabled")) -> ()  [unwired: 2 in, 2 out]
                n202 = property on="TEC Connect" class="Bool"("DisabledEnum"=T6."Disabled and Grayed Out" ("Disabled")) -> ()  [unwired: 2 in, 2 out]
              }
            }
          }
        }
      }
      event "TEC Auto-Detect": Value Change {
        n203 = event-data() -> ("NewVal"=w354:bool)  [unwired: 1 in, 5 out]
        n204 = Boolean To (0,1)(Boolean=w354) -> (0, 1=w352:i16)
        n205 = To Double Precision Float(number=w352) -> (double precision float=w351:dbl)
        n206 = Bundle By Name(cluster=w356, "Message"=TEC_Queue_Messages."Auto Detect", "Data"=w351) -> (w353:cluster{"Message":T4, "TEC ID":i32, "Data":dbl})
        n207 = Enqueue Element(queue=w357, element=w353) -> ()  [unwired: 2 in, 3 out]
      }
      event "TEC Connect": Value Change {
        n208 = event-data() -> ("NewVal"=w363:bool)  [unwired: 1 in, 5 out]
        n209 = Boolean To (0,1)(Boolean=w363) -> (0, 1=w361:i16)
        n210 = To Double Precision Float(number=w361) -> (double precision float=w360:dbl)
        n211 = Bundle By Name(cluster=w365, "Message"=TEC_Queue_Messages."Connect", "TEC ID"="TEC Address", "Data"=w360) -> (w362:cluster{"Message":T4, "TEC ID":i32, "Data":dbl})
        n212 = Enqueue Element(queue=w366, element=w362) -> ()  [unwired: 2 in, 3 out]
      }
      event "TEC Disconnect": Value Change {
        n213 = event-data() -> ("NewVal"=w372:bool)  [unwired: 1 in, 5 out]
        n214 = property on="TEC Address" class="Ring (strict)"() -> ("Value"=w368:u16)  [unwired: 2 in, 2 out]
        n215 = Boolean To (0,1)(Boolean=w372) -> (0, 1=w370:i16)
        n216 = To Double Precision Float(number=w370) -> (double precision float=w369:dbl)
        n217 = Bundle By Name(cluster=w374, "Message"=TEC_Queue_Messages."Disconnect", "TEC ID"=w368, "Data"=w369) -> (w371:cluster{"Message":T4, "TEC ID":i32, "Data":dbl})
        n218 = Enqueue Element(queue=w375, element=w371) -> ()  [unwired: 2 in, 3 out]
      }
      event "LED Connect": Value Change {
        n219 = event-data() -> ("NewVal"=w383:bool)  [unwired: 1 in, 5 out]
        n220 = Boolean To (0,1)(Boolean=w383) -> (0, 1=w382:i16)
        n221 = To Double Precision Float(number=w382) -> (double precision float=w380:dbl)
        n222 = Bundle By Name(cluster=w381, "Message"=LED_Controller_Messages."Connect", "Data"=w380) -> (w378:cluster{"Message":T5, "Data":dbl})
        n223 = Enqueue Element(queue=w379, element=w378) -> ()  [unwired: 2 in, 3 out]
      }
      event "LED Auto-Connect": Value Change {
        n224 = event-data() -> ("NewVal"=w387:bool)  [unwired: 1 in, 5 out]
        n225 = case shown="True" w387 {
          tunnel: w386 -> [_ w394]
          tunnel: w385 -> [_ w393]
          frame False {
            n226 = property on="LED Controller Status" class="Bool (strict)"() -> ("Value"=w388:bool)  [unwired: 2 in, 2 out]
            n227 = case shown="False" w388 {
              frame True {
                n228 = property on="LED Disconnect" class="Bool"("DisabledEnum"=T6."Enabled" ("Disabled")) -> ()  [unwired: 2 in, 2 out]
                n229 = property on="LED Connect" class="Bool"("DisabledEnum"=T6."Disabled and Grayed Out" ("Disabled")) -> ()  [unwired: 2 in, 2 out]
              }
              frame False {
                n230 = property on="LED Disconnect" class="Bool"("DisabledEnum"=T6."Disabled and Grayed Out" ("Disabled")) -> ()  [unwired: 2 in, 2 out]
                n231 = property on="LED Connect" class="Bool"("DisabledEnum"=T6."Enabled" ("Disabled")) -> ()  [unwired: 2 in, 2 out]
              }
            }
          }
          frame True {
            n232 = property on="LED Controller Status" class="Bool (strict)"() -> ("Value"=w395:bool)  [unwired: 2 in, 2 out]
            n233 = case shown="False" w395 {
              tunnel: w394 -> [w400 _]
              tunnel: w393 -> [w399 _]
              frame False {
                n234 = Boolean To (0,1)(Boolean=TRUE) -> (0, 1=w404:i16)
                n235 = To Double Precision Float(number=w404) -> (double precision float=w403:dbl)
                n236 = Bundle By Name(cluster=w399, "Message"=LED_Controller_Messages."Connect", "Data"=w403) -> (w402:cluster{"Message":T5, "Data":dbl})
                n237 = Enqueue Element(queue=w400, element=w402) -> ()  [unwired: 2 in, 3 out]
              }
              frame True {
              }
            }
            n238 = property on="LED Disconnect" class="Bool"("DisabledEnum"=T6."Disabled and Grayed Out" ("Disabled")) -> ()  [unwired: 2 in, 2 out]
            n239 = property on="LED Connect" class="Bool"("DisabledEnum"=T6."Disabled and Grayed Out" ("Disabled")) -> ()  [unwired: 2 in, 2 out]
          }
        }
      }
      event "TEC Auto-Connect": Value Change {
        n240 = event-data() -> ("NewVal"=w408:bool)  [unwired: 1 in, 5 out]
        n241 = case shown="True" w408 {
          tunnel: w407 -> [_ w419]
          tunnel: w406 -> [_ w418]
          frame False {
            n242 = property on="TEC Address" class="Ring (strict)"("DisabledEnum"=T6."Enabled" ("Disabled")) -> (error out=w410:errorcluster)  [unwired: 2 in, 1 out]
            n243 = property on="TEC Address" class="Ring (strict)"(error in=w410) -> (error out=w409:errorcluster, "Value"=w411:u16)  [unwired: 1 in, 1 out]
            n244 = property on="TEC Address" class="Ring (strict)"(error in=w409, "Val(Sgnl)"=w411) -> ()  [unwired: 1 in, 2 out]
          }
          frame True {
            w417 = T6."Disabled and Grayed Out" ("Disabled")
            n245 = property on="TEC COM Status" class="Arr (strict)"() -> ("Value"=w416:bool[])  [unwired: 2 in, 2 out]
            n246 = Not(x=w416) -> (.not. x?=w415:bool[])
            n247 = Boolean Array To Number(Boolean array=w415) -> (number=w413:u32)
            n248 = Equal To 0?(x=w413) -> (x = 0?=w414:bool)
            n249 = case shown="False" w414 {
              tunnel: w419 -> [w423 _]
              tunnel: w418 -> [w422 _]
              frame False {
                n250 = Bundle By Name(cluster=w422, "Message"=TEC_Queue_Messages."Connect", "TEC ID"=0) -> (w424:cluster{"Message":T4, "TEC ID":i32, "Data":dbl})
                n251 = Enqueue Element(queue=w423, element=w424) -> ()  [unwired: 2 in, 3 out]
              }
              frame True {
              }
            }
            n252 = property on="TEC Address" class="Ring (strict)"("DisabledEnum"=w417) -> ()  [unwired: 2 in, 2 out]
            n253 = property on="TEC Disconnect" class="Bool"("DisabledEnum"=w417) -> ()  [unwired: 2 in, 2 out]
            n254 = property on="TEC Connect" class="Bool"("DisabledEnum"=w417) -> ()  [unwired: 2 in, 2 out]
          }
        }
      }
      event "LED Disconnect": Value Change {
        n255 = event-data() -> ("NewVal"=w432:bool)  [unwired: 1 in, 5 out]
        n256 = Boolean To (0,1)(Boolean=w432) -> (0, 1=w431:i16)
        n257 = To Double Precision Float(number=w431) -> (double precision float=w429:dbl)
        n258 = Bundle By Name(cluster=w430, "Message"=LED_Controller_Messages."Disconnect", "Data"=w429) -> (w427:cluster{"Message":T5, "Data":dbl})
        n259 = Enqueue Element(queue=w428, element=w427) -> ()  [unwired: 2 in, 3 out]
      }
    }
  }
  n260 = while {
    tunnel: w17 -> [w434]
    shift-right: [w443] -> _
    shift-left: _ -> [w442]
    tunnel: w7 -> [w440]
    shift-right: [w438] -> _
    shift-left: T3 {"MODE A"=FALSE, "MODE B"=FALSE, "RANGE A"=FALSE, "RANGE B"=FALSE} -> [w439]
    tunnel: [w433] -> _
    stop <- w441 stop-if-true
    # "LED Controller Functions"
    n261 = Dequeue Element(queue=w434, timeout in ms (-1)="LED monitor\nperiod (ms)", error in (no error)=w440) -> (element=w444:cluster{"Message":T5, "Data":dbl}, timed out?=w445:bool)  [unwired: 2 out]
    n262 = case shown="False" w445 {
      tunnel: w444 -> [w459 _]
      tunnel: [w457 w584] -> w443
      tunnel: w442 -> [w456 w614]
      tunnel: [w455 _] -> w441
      tunnel: w434 -> [w453 _]
      tunnel: [w452 w601] -> w437
      tunnel: w439 -> [w451 w600]
      tunnel: [w450 w600] -> w438
      frame False {
        n263 = Unbundle By Name(w459) -> ("Message"=w458:T5, "Data"=w454:dbl)
        n264 = case shown="\"Set Range A\"" w458 {
          tunnel: [w464 refnum<visa-resource-name> refnum ("VISA Refnum out") refnum<visa-resource-name> refnum ("VISA Refnum out") w506 w517 w526 w537 w547 w559] -> w457
          tunnel: w456 -> [_ w488 w491 w508 w519 w527 w538 w553 w565]
          tunnel: [_ _ TRUE _ _ _ _ _ _] -> w455
          tunnel: w454 -> [_ _ _ w507 w518 w530 w541 w549 w561]
          tunnel: w453 -> [w463 _ _ _ _ _ _ _ _]
          tunnel: [w462 FALSE FALSE w500 w511 w522 w533 w542 w554] -> w452
          tunnel: w451 -> [w461 w485 w489 w504 w515 w528 w539 w546 w558]
          tunnel: [w461 w485 w489 w505 w516 w529 w540 w546 w558] -> w450
          frame "Connect", Default {
            n265 = call "PAS_open_serial.vi"("VISA Refnum in"="LED Controller COM Port") -> ("error out"=w466:errorcluster, "VISA Refnum out"=w465:refnum<visa-resource-name>)  [unwired: 9 in]
            n266 = case shown="No Error" w466 {
              tunnel: w465 -> [w470 _]
              tunnel: [w470 refnum<visa-resource-name> refnum ("VISA Refnum out")] -> w464
              tunnel: w463 -> [_ w478]
              tunnel: [TRUE FALSE] -> w462
              tunnel: "LED Auto-Connect" -> [w468 w475]
              frame No Error {
                n267 = case shown="True" w468 {
                  frame False {
                    n268 = property on="LED Disconnect" class="Bool"("DisabledEnum"=T6."Enabled" ("Disabled")) -> ()  [unwired: 2 in, 2 out]
                    n269 = property on="LED Connect" class="Bool"("DisabledEnum"=T6."Disabled and Grayed Out" ("Disabled")) -> ()  [unwired: 2 in, 2 out]
                  }
                  frame True {
                    n270 = property on="LED Disconnect" class="Bool"("DisabledEnum"=T6."Disabled and Grayed Out" ("Disabled")) -> ()  [unwired: 2 in, 2 out]
                    n271 = property on="LED Connect" class="Bool"("DisabledEnum"=T6."Disabled and Grayed Out" ("Disabled")) -> ()  [unwired: 2 in, 2 out]
                  }
                }
              }
              frame Error {
                n272 = case shown="True" w475 {
                  tunnel: w478 -> [_ w482]
                  frame False {
                  }
                  frame True {
                    w481 = cluster{"Message":T5, "Data":dbl} {"Message"=enum."Set Output B", "Data"=0.0}  # LED
                    n273 = Bundle By Name(cluster=w481, "Message"=LED_Controller_Messages."Connect") -> (w479:cluster{"Message":T5, "Data":dbl})
                    n274 = Enqueue Element(queue=w482, element=w479) -> ()  [unwired: 2 in, 3 out]
                  }
                }
              }
            }
          }
          frame "Disconnect" {
            n275 = VISA Close(VISA resource name=w488) -> ()  [unwired: 1 in, 1 out]
            n276 = property on="LED Disconnect" class="Bool"("DisabledEnum"=T6."Disabled and Grayed Out" ("Disabled")) -> ()  [unwired: 2 in, 2 out]
            n277 = property on="LED Connect" class="Bool"("DisabledEnum"=T6."Enabled" ("Disabled")) -> ()  [unwired: 2 in, 2 out]
          }
          frame "Exit" {
            n278 = Not Equal?(x=refnum<visa-resource-name> refnum ("VISA Refnum out"), y=w491) -> (x != y?=w492:bool)
            n279 = case shown="True" w492 {
              tunnel: w491 -> [_ w497]
              frame False {
              }
              frame True {
                n280 = VISA Close(VISA resource name=w497) -> (error out=w496:errorcluster)  [unwired: 1 in]
                n281 = call <vilib>:"Clear Errors.vi"("error in (no error)"=w496) -> ()  [unwired: 5 in, 2 out]
              }
            }
          }
          frame "Set Mode A" {
            # "wires reversed to match wiring in control box"
            n282 = Not Equal To 0?(x=w507) -> (x != 0?=w498:bool)
            n283 = Unbundle By Name(w504) -> ("MODE B"=w499:bool)
            n284 = Bundle By Name(cluster=w504, "MODE A"=w498) -> (w505:T3)
            n285 = call "PAS_set_regulation_mode.vi"("MODE B"=w498, "MODE A"=w499, "VISA Refnum in"=w508) -> ("error out"=w502:errorcluster, "Success?"=w501:bool, "VISA Refnum out"=w506:refnum<visa-resource-name>)  [unwired: 6 in]
            n286 = Unbundle(w502) -> ("status"=w503:bool)  [unwired: 2 out]
            n287 = Compound Arithmetic op=AND(w501, invert w503) -> (w500:bool)
          }
          frame "Set Mode B" {
            # "wires reversed to match wiring in control box"
            n288 = Not Equal To 0?(x=w518) -> (x != 0?=w509:bool)
            n289 = Unbundle By Name(w515) -> ("MODE A"=w510:bool)
            n290 = Bundle By Name(cluster=w515, "MODE B"=w509) -> (w516:T3)
            n291 = call "PAS_set_regulation_mode.vi"("MODE B"=w510, "MODE A"=w509, "VISA Refnum in"=w519) -> ("error out"=w513:errorcluster, "Success?"=w512:bool, "VISA Refnum out"=w517:refnum<visa-resource-name>)  [unwired: 6 in]
            n292 = Unbundle(w513) -> ("status"=w514:bool)  [unwired: 2 out]
            n293 = Compound Arithmetic op=AND(w512, invert w514) -> (w511:bool)
          }
          frame "Set Range A" {
            # "wires reversed to match wiring in control box"
            n294 = Not Equal To 0?(x=w530) -> (x != 0?=w520:bool)
            n295 = Unbundle By Name(w528) -> ("RANGE B"=w521:bool)
            n296 = Bundle By Name(cluster=w528, "RANGE A"=w520) -> (w529:T3)
            n297 = call "PAS_set_regulation_range.vi"("Range B"=w520, "Range A"=w521, "VISA Refnum in"=w527) -> ("error out"=w524:errorcluster, "Success?"=w523:bool, "VISA Refnum out"=w526:refnum<visa-resource-name>)  [unwired: 6 in]
            n298 = Unbundle(w524) -> ("status"=w525:bool)  [unwired: 2 out]
            n299 = Compound Arithmetic op=AND(w523, invert w525) -> (w522:bool)
          }
          frame "Set Range B" {
            # "wires reversed to match wiring in control box"
            n300 = Not Equal To 0?(x=w541) -> (x != 0?=w532:bool)
            n301 = Unbundle By Name(w539) -> ("RANGE A"=w531:bool)
            n302 = Bundle By Name(cluster=w539, "RANGE B"=w532) -> (w540:T3)
            n303 = call "PAS_set_regulation_range.vi"("Range B"=w531, "Range A"=w532, "VISA Refnum in"=w538) -> ("error out"=w535:errorcluster, "Success?"=w534:bool, "VISA Refnum out"=w537:refnum<visa-resource-name>)  [unwired: 6 in]
            n304 = Unbundle(w535) -> ("status"=w536:bool)  [unwired: 2 out]
            n305 = Compound Arithmetic op=AND(w534, invert w536) -> (w533:bool)
          }
          frame "Set Output A" {
            w550 = u16 1 items=["CH 1"=1, "CH 2"=2, "BOTH"=3] ("Channel")
            w551 = u16 0 items=["DAC", "ADC 1 (temp)", "ADC 2", "ADC 3"] ("Channel")
            n306 = call "PAS_set_channel.vi"("Channel"=w551, "VISA Refnum in"=w553) -> ("error out"=w548:errorcluster, "VISA Refnum out"=w552:refnum<visa-resource-name>)  [unwired: 7 in, 1 out]
            n307 = call "PAS_set_DAC.vi"("error in (no error)"=w548, "Voltage"=w549, "Channel"=w550, "VISA Refnum in"=w552) -> ("error out"=w544:errorcluster, "Success?"=w543:bool, "VISA Refnum out"=w547:refnum<visa-resource-name>)  [unwired: 5 in]
            n308 = Unbundle(w544) -> ("status"=w545:bool)  [unwired: 2 out]
            n309 = Compound Arithmetic op=AND(w543, invert w545) -> (w542:bool)
          }
          frame "Set Output B" {
            w562 = u16 2 items=["CH 1"=1, "CH 2"=2, "BOTH"=3] ("Channel")
            w563 = u16 0 items=["DAC", "ADC 1 (temp)", "ADC 2", "ADC 3"] ("Channel")
            n310 = call "PAS_set_channel.vi"("Channel"=w563, "VISA Refnum in"=w565) -> ("error out"=w560:errorcluster, "VISA Refnum out"=w564:refnum<visa-resource-name>)  [unwired: 7 in, 1 out]
            n311 = call "PAS_set_DAC.vi"("error in (no error)"=w560, "Voltage"=w561, "Channel"=w562, "VISA Refnum in"=w564) -> ("error out"=w557:errorcluster, "Success?"=w555:bool, "VISA Refnum out"=w559:refnum<visa-resource-name>)  [unwired: 5 in]
            n312 = Unbundle(w557) -> ("status"=w556:bool)  [unwired: 2 out]
            n313 = Compound Arithmetic op=AND(w555, invert w556) -> (w554:bool)
          }
        }
      }
      frame True {
        w608 = u16 2 items=["DAC", "ADC 1 (temp)", "ADC 2", "ADC 3"] ("Channel")
        w609 = u16 3 items=["DAC", "ADC 1 (temp)", "ADC 2", "ADC 3"] ("Channel")
        w613 = u16 1 items=["DAC", "ADC 1 (temp)", "ADC 2", "ADC 3"] ("Channel")
        n314 = property on="Low Light Offset B" class="DigNum (strict)"() -> ("Value"=w582:dbl)  [unwired: 2 in, 2 out]
        n315 = property on="High Light Offset B" class="DigNum (strict)"() -> ("Value"=w583:dbl)  [unwired: 2 in, 2 out]
        n316 = call "PAS_set_channel.vi"("Channel"=w613, "VISA Refnum in"=w614) -> ("error out"=w588:errorcluster, "VISA Refnum out"=w591:refnum<visa-resource-name>)  [unwired: 7 in, 1 out]
        n317 = Unbundle By Name(w600) -> ("RANGE B"=w579:bool, "RANGE A"=w578:bool)
        n318 = Select(t=w583, s=w579, f=w582) -> (s? t:f=w574:dbl)
        n319 = call "PAS_read_voltage.vi"("error in (no error)"=w588, "Hi-res Mode"=FALSE ("Hi-res mode"), "VISA Refnum in"=w591) -> ("error out"=w589:errorcluster, "voltage (double)"=w567:dbl, "VISA Refnum out"=w590:refnum<visa-resource-name>)  [unwired: 5 in, 1 out]
        "LED Driver Ground Offset (mV)" <- w567
        n320 = call "PAS_set_channel.vi"("error in (no error)"=w589, "Channel"=w609, "VISA Refnum in"=w590) -> ("error out"=w610:errorcluster, "VISA Refnum out"=w611:refnum<visa-resource-name>)  [unwired: 6 in, 1 out]
        n321 = call "PAS_read_voltage.vi"("error in (no error)"=w610, "Hi-res Mode"=FALSE, "VISA Refnum in"=w611) -> ("error out"=w603:errorcluster, "voltage (double)"=w572:dbl, "VISA Refnum out"=w604:refnum<visa-resource-name>)  [unwired: 5 in, 1 out]
        "Diode Raw B" <- w572
        n322 = call "PAS_set_channel.vi"("error in (no error)"=w603, "Channel"=w608, "VISA Refnum in"=w604) -> ("error out"=w607:errorcluster, "VISA Refnum out"=w606:refnum<visa-resource-name>)  [unwired: 6 in, 1 out]
        n323 = call "PAS_read_voltage.vi"("error in (no error)"=w607, "Hi-res Mode"=FALSE, "VISA Refnum in"=w606) -> ("error out"=w586:errorcluster, "voltage (double)"=w566:dbl, "VISA Refnum out"=w584:refnum<visa-resource-name>)  [unwired: 5 in, 1 out]
        "Diode Raw A" <- w566
        n324 = case shown="True" "Dynamic Offset Cor." {
          tunnel: w586 -> [w615 w621]
          tunnel: [w615 w620] -> w585
          tunnel: w567 -> [_ w618]
          tunnel: w584 -> [_ w616]
          frame False {
          }
          frame True {
            w623 = u16 2 items=["CH 1"=1, "CH 2"=2, "BOTH"=3] ("Channel")
            w624 = u16 0 items=["DAC", "ADC 1 (temp)", "ADC 2", "ADC 3"] ("Channel")
            n325 = property on="Light level raw B" class="DigNum (strict)"() -> ("Value"=w619:dbl)  [unwired: 2 in, 2 out]
            n326 = Add(x=w618, y=w619) -> (x+y=w617:dbl)
            n327 = call "PAS_set_channel.vi"("error in (no error)"=w621, "Channel"=w624, "VISA Refnum in"=w616) -> ("error out"=w622:errorcluster, "VISA Refnum out"=w625:refnum<visa-resource-name>)  [unwired: 6 in, 1 out]
            n328 = call "PAS_set_DAC.vi"("error in (no error)"=w622, "Voltage"=w617, "Channel"=w623, "VISA Refnum in"=w625) -> ("error out"=w620:errorcluster)  [unwired: 5 in, 2 out]
          }
        }
        n329 = Select(t=w567, s=TRUE, f=0.0 ("y")) -> (s? t:f=w570:dbl)
        n330 = Subtract(x=w572, y=w570) -> (x-y=w573:dbl)
        n331 = property on="High Light 1 Sun Level A" class="DigNum (strict)"() -> ("Value"=w597:dbl)  [unwired: 2 in, 2 out]
        n332 = property on="Low Light 1 Sun Level A" class="DigNum (strict)"() -> ("Value"=w596:dbl)  [unwired: 2 in, 2 out]
        n333 = property on="High Light 1 Sun Level B" class="DigNum (strict)"() -> ("Value"=w598:dbl)  [unwired: 2 in, 2 out]
        n334 = property on="Low Light 1 Sun Level B" class="DigNum (strict)"() -> ("Value"=w599:dbl)  [unwired: 2 in, 2 out]
        n335 = Subtract(x=w573, y=w574) -> (x-y=w575:dbl)
        n336 = Unbundle By Name(w585) -> ("status"=w602:bool)
        n337 = Select(t=w597, s=w578, f=w596) -> (s? t:f=w595:dbl)
        n338 = Select(t=w598, s=w579, f=w599) -> (s? t:f=w594:dbl)
        n339 = property on="Low Light Offset A" class="DigNum (strict)"() -> ("Value"=w580:dbl)  [unwired: 2 in, 2 out]
        n340 = property on="High Light Offset A" class="DigNum (strict)"() -> ("Value"=w581:dbl)  [unwired: 2 in, 2 out]
        n341 = Not(x=w602) -> (.not. x?=w601:bool)
        n342 = Divide(x=w575, y=w594) -> (x/y=→"Light Level B" →"Light Level Monitor B":dbl)
        n343 = Select(t=w581, s=w578, f=w580) -> (s? t:f=w576:dbl)
        n344 = Subtract(x=w566, y=w576) -> (x-y=w577:dbl)
        n345 = Divide(x=w577, y=w595) -> (x/y=→"Light Level A" →"Light Level Monitor A":dbl)
      }
    }
    "LED Controller Status" <- w437
    n346 = property on="LED Auto-Connect" class="Bool (strict)"() -> ("Value"=w436:bool)  [unwired: 2 in, 2 out]
    n347 = Compound Arithmetic op=AND(invert w437, w436) -> (w435:bool)
    n348 = case shown="True" w435 {
      tunnel: w434 -> [_ w449]
      tunnel: [errorcluster {"status"=FALSE, "code"=0, "source"=""} ("error out") w448] -> w433
      frame False {
      }
      frame True {
        n349 = call "LED COM Reconnect.vi"("Queue in"=w449) -> ("error out"=w448:errorcluster)  [unwired: 10 in]
      }
    }
  }
  n350 = property on="TimingList2" class="MCListbox (strict)"() -> ("ItemNames"=w2:string[][])  [unwired: 2 in, 2 out]
  n351 = property on="TimingList1" class="MCListbox (strict)"() -> ("ItemNames"=w5:string[][])  [unwired: 2 in, 2 out]
  n352 = Fract/Exp String To Number(string=w2) -> (number=w1:dbl[][])  [unwired: 3 in, 1 out]
  n353 = Fract/Exp String To Number(string=w5) -> (number=w4:dbl[][])  [unwired: 3 in, 1 out]
  n354 = local write "ControlTable2"(w1) -> ()
  n355 = local write "ControlTable1"(w4) -> ()
  n356 = local write "stopped"(FALSE ("stopped")) -> ()
  n357 = while {
    stop <- w639 stop-if-true
    n358 = local read "Automatic Control Active H1"() -> (w641:bool)
    n359 = case shown="False" w641 {
      frame False {
        n360 = global write "StartStopPause.vi" "StartStopPauseArray1"(bool[][] [[FALSE, FALSE, FALSE], [FALSE, FALSE, FALSE], [FALSE, FALSE, FALSE], [FALSE, FALSE, FALSE], [FALSE, FALSE, FALSE], [FALSE, FALSE, FALSE], [FALSE, FALSE, FALSE], [FALSE, FALSE, FALSE]] ("StartStopPauseArray2")) -> ()
      }
      frame True {
        n361 = local read "started last"() -> (w722:timestamp)
        n362 = local read "ControlTable1"() -> (w720:dbl[][])
        n363 = Get Date/Time In Seconds() -> (seconds since 1Jan1904=w723:timestamp)
        n364 = local read "started at"() -> (w725:timestamp)
        n365 = Subtract(x=w723, y=w725) -> (x-y=→"ElapsedTime":dbl)
        n366 = local read "Active Row"() -> (w715:i32)
        n367 = Subtract(x=w723, y=w722) -> (x-y=w721:dbl)
        "Current Row" <- w721
        n368 = Index Array(array=w720, index (row)=w715, index (col)=0 ("disabled index (col)")) -> (element=w719:dbl)
        n369 = Multiply(x=w719, y=3600.0) -> (x*y=w718:dbl)
        n370 = Equal?(x=w715, y=-1) -> (x = y?=w714:bool)
        n371 = Greater?(x=w721, y=w718) -> (0:w716:bool)
        n372 = Or(x=w716, y=w714) -> (x .or. y?=w712:bool)
        n373 = case shown="True" w712 {
          tunnel: w715 -> [_ w746]
          tunnel: w720 -> [_ w730]
          frame False {
          }
          frame True {
            n374 = Increment(x=w746) -> (x+1=w741:i32)
            n375 = Array Size(array=w730) -> (size(s)=w744:i32[])
            n376 = Index Array(array=w744) -> (element=w743:i32)  [unwired: 1 in]
            n377 = Greater Or Equal?(x=w741, y=w743) -> (x >= y?=w742:bool)
            n378 = case shown="True" w742 {
              tunnel: [w773 "loop to row"] -> w729
              tunnel: w741 -> [w773 _]
              frame False {
              }
              frame True {
              }
            }
            n379 = local write "TimingList1"(w729) -> ()
            n380 = local write "Active Row"(w729) -> ()
            n381 = Index Array(array=w730, index (row)=w729) -> (element=w754:dbl[])  [unwired: 1 in]
            n382 = Index Array(array=w754) -> (element #2=w748:dbl, element #3=w753:dbl, element #4=w752:dbl, element #5=w751:dbl, element #6=w750:dbl, element #7=w740:dbl, element #8=w738:dbl, element #9=w737:dbl)  [unwired: 9 in, 1 out]
            n383 = for {
              N: 8 -> [_]
              shift-right: [w771] -> _
              shift-left: w740 -> [w770]
              tunnel: [w765] -> w736 mode=indexing
              shift-right: [w756] -> _
              shift-left: w738 -> [w769]
              tunnel: [w757] -> w735 mode=indexing
              shift-right: [w760] -> _
              shift-left: w737 -> [w766]
              tunnel: [w759] -> w734 mode=indexing
              n384 = Quotient & Remainder(x=w770, y=10.0) -> (x-y*floor(x/y)=w764:dbl, floor(x/y)=w771:dbl)
              n385 = Quotient & Remainder(x=w769, y=10.0) -> (x-y*floor(x/y)=w755:dbl, floor(x/y)=w756:dbl)
              n386 = Quotient & Remainder(x=w766, y=10.0) -> (x-y*floor(x/y)=w758:dbl, floor(x/y)=w760:dbl)
              n387 = Equal?(x=w764, y=1.0) -> (x = y?=w765:bool)
              n388 = Equal?(x=w758, y=1.0) -> (x = y?=w759:bool)
              n389 = Equal?(x=w755, y=1.0) -> (x = y?=w757:bool)
            }
            n390 = Greater?(x=w748, y=0.08) -> (0:w749:bool)
            n391 = property on="Light Range A" class="Bool (strict)"("Value"=w749, "Val(Sgnl)"=w749) -> ()  [unwired: 2 in, 2 out]
            n392 = Get Date/Time In Seconds() -> (seconds since 1Jan1904=→"started last":timestamp)
            n393 = Reverse 1D Array(array=w736) -> (reversed array=w733:bool[])
            n394 = Reverse 1D Array(array=w735) -> (reversed array=w731:bool[])
            n395 = Reverse 1D Array(array=w734) -> (reversed array=w732:bool[])
            n396 = property on="Light Level set A" class="Slide (strict)"("Value"=w748, "Val(Sgnl)"=w748) -> ()  [unwired: 2 in, 2 out]
            n397 = property on="cell 4A set" class="DigNum (strict)"("Value"=w750, "Val(Sgnl)"=w750) -> ()  [unwired: 2 in, 2 out]
            n398 = property on="cell 1A set" class="DigNum (strict)"("Value"=w753, "Val(Sgnl)"=w753) -> ()  [unwired: 2 in, 2 out]
            n399 = property on="cell 2A set" class="DigNum (strict)"("Value"=w752, "Val(Sgnl)"=w752) -> ()  [unwired: 2 in, 2 out]
            n400 = property on="cell 3A set" class="DigNum (strict)"("Value"=w751, "Val(Sgnl)"=w751) -> ()  [unwired: 2 in, 2 out]
            n401 = Build Array(w733, w731, w732) -> (w728:bool[][])
            n402 = Transpose 2D Array(2D array=w728) -> (transposed array=w727:bool[][])
            n403 = global write "StartStopPause.vi" "StartStopPauseArray1"(w727) -> ()
          }
        }
      }
    }
    n404 = local read "Automatic Control Active H2"() -> (w627:bool)
    n405 = case shown="False" w627 {
      frame False {
        n406 = global write "StartStopPause.vi" "StartStopPauseArray2"(bool[][] [[FALSE, FALSE, FALSE], [FALSE, FALSE, FALSE], [FALSE, FALSE, FALSE], [FALSE, FALSE, FALSE], [FALSE, FALSE, FALSE], [FALSE, FALSE, FALSE], [FALSE, FALSE, FALSE], [FALSE, FALSE, FALSE]] ("StartStopPauseArray2")) -> ()
      }
      frame True {
        n407 = local read "started last 2"() -> (w654:timestamp)
        n408 = local read "ControlTable2"() -> (w652:dbl[][])
        n409 = Get Date/Time In Seconds() -> (seconds since 1Jan1904=w655:timestamp)
        n410 = local read "started at 2"() -> (w643:timestamp)
        n411 = Subtract(x=w655, y=w643) -> (x-y=→"ElapsedTime 2":dbl)
        n412 = local read "Active Row 2"() -> (w647:i32)
        n413 = Subtract(x=w655, y=w654) -> (x-y=w653:dbl)
        "Current Row 2" <- w653
        n414 = Index Array(array=w652, index (row)=w647, index (col)=0 ("disabled index (col)")) -> (element=w651:dbl)
        n415 = Multiply(x=w651, y=3600.0) -> (x*y=w650:dbl)
        n416 = Equal?(x=w647, y=-1) -> (x = y?=w646:bool)
        n417 = Greater?(x=w653, y=w650) -> (0:w648:bool)
        n418 = Or(x=w648, y=w646) -> (x .or. y?=w644:bool)
        n419 = case shown="True" w644 {
          tunnel: w647 -> [_ w683]
          tunnel: w652 -> [_ w667]
          frame False {
          }
          frame True {
            n420 = Increment(x=w683) -> (x+1=w678:i32)
            n421 = Array Size(array=w667) -> (size(s)=w681:i32[])
            n422 = Index Array(array=w681) -> (element=w680:i32)  [unwired: 1 in]
            n423 = Greater Or Equal?(x=w678, y=w680) -> (x >= y?=w679:bool)
            n424 = case shown="True" w679 {
              tunnel: [w704 "loop to row 2"] -> w666
              tunnel: w678 -> [w704 _]
              frame False {
              }
              frame True {
              }
            }
            n425 = local write "TimingList2"(w666) -> ()
            n426 = local write "Active Row 2"(w666) -> ()
            n427 = Index Array(array=w667, index (row)=w666) -> (element=w685:dbl[])  [unwired: 1 in]
            n428 = Index Array(array=w685) -> (element #2=w663:dbl, element #3=w662:dbl, element #4=w661:dbl, element #5=w660:dbl, element #6=w659:dbl, element #7=w677:dbl, element #8=w675:dbl, element #9=w674:dbl)  [unwired: 9 in, 1 out]
            n429 = for {
              N: 8 -> [_]
              shift-right: [w702] -> _
              shift-left: w677 -> [w701]
              tunnel: [w696] -> w673 mode=indexing
              shift-right: [w687] -> _
              shift-left: w675 -> [w700]
              tunnel: [w688] -> w672 mode=indexing
              shift-right: [w691] -> _
              shift-left: w674 -> [w697]
              tunnel: [w690] -> w671 mode=indexing
              n430 = Quotient & Remainder(x=w701, y=10.0) -> (x-y*floor(x/y)=w695:dbl, floor(x/y)=w702:dbl)
              n431 = Quotient & Remainder(x=w700, y=10.0) -> (x-y*floor(x/y)=w686:dbl, floor(x/y)=w687:dbl)
              n432 = Quotient & Remainder(x=w697, y=10.0) -> (x-y*floor(x/y)=w689:dbl, floor(x/y)=w691:dbl)
              n433 = Equal?(x=w695, y=1.0) -> (x = y?=w696:bool)
              n434 = Equal?(x=w689, y=1.0) -> (x = y?=w690:bool)
              n435 = Equal?(x=w686, y=1.0) -> (x = y?=w688:bool)
            }
            n436 = Greater?(x=w663, y=0.08) -> (0:w658:bool)
            n437 = property on="Light Range B" class="Bool (strict)"("Value"=w658, "Val(Sgnl)"=w658) -> ()  [unwired: 2 in, 2 out]
            n438 = Get Date/Time In Seconds() -> (seconds since 1Jan1904=→"started last 2":timestamp)
            n439 = Reverse 1D Array(array=w673) -> (reversed array=w670:bool[])
            n440 = Reverse 1D Array(array=w672) -> (reversed array=w668:bool[])
            n441 = Reverse 1D Array(array=w671) -> (reversed array=w669:bool[])
            n442 = property on="Light Level set B" class="Slide (strict)"("Value"=w663, "Val(Sgnl)"=w663) -> ()  [unwired: 2 in, 2 out]
            n443 = property on="cell 3B set" class="DigNum (strict)"("Value"=w660, "Val(Sgnl)"=w660) -> ()  [unwired: 2 in, 2 out]
            n444 = property on="cell 4B set" class="DigNum (strict)"("Value"=w659, "Val(Sgnl)"=w659) -> ()  [unwired: 2 in, 2 out]
            n445 = property on="cell 1B set" class="DigNum (strict)"("Value"=w662, "Val(Sgnl)"=w662) -> ()  [unwired: 2 in, 2 out]
            n446 = property on="cell 2B set" class="DigNum (strict)"("Value"=w661, "Val(Sgnl)"=w661) -> ()  [unwired: 2 in, 2 out]
            n447 = Build Array(w670, w668, w669) -> (w665:bool[][])
            n448 = Transpose 2D Array(2D array=w665) -> (transposed array=w664:bool[][])
            n449 = global write "StartStopPause.vi" "StartStopPauseArray2"(w664) -> ()
          }
        }
      }
    }
    n450 = local read "Light Level A"() -> (w637:dbl)
    n451 = local read "Light Level B"() -> (w636:dbl)
    n452 = local read "TempArray"() -> (w633:dbl[])
    n453 = for {
      tunnel: w633 -> [w707] mode=indexing
      shift-right: [w706] -> w630
      shift-left: dbl[] [] -> [w708]
      n454 = Insert Into Array(array=w708, new element #1=w707, new element #2=w707) -> (w706:dbl[])  [unwired: 1 in]
    }
    n455 = for {
      N: 8 -> [_]
      tunnel: [w710] -> w635 mode=indexing
      tunnel: w637 -> [w710]
      tunnel: [w709] -> w634 mode=indexing
      tunnel: w636 -> [w709]
    }
    n456 = Insert Into Array(array=w635, new element=w634) -> (w631:dbl[])  [unwired: 1 in]
    n457 = global read "StartStopPause.vi" "StartStopPauseArray1"() -> (→"StartStopPauseArray1":bool[][])
    n458 = global read "StartStopPause.vi" "StartStopPauseArray2"() -> (→"StartStopPauseArray2":bool[][])
    n459 = Build Array(w631, w630) -> (w629:dbl[][])
    n460 = global write "IntensityTemperature.vi" "IntTemp"(w629) -> ()
    n461 = local read "stopped"() -> (w639:bool)
    n462 = Wait Until Next ms Multiple(millisecond multiple=u32 200) -> ()  [unwired: 1 out]
  }
  n463 = while {
    tunnel: w21 -> [w776]
    shift-right: [w789] -> _
    shift-left: refnum<visa-resource-name>[] [] ("TEC COM Ports") -> [w788]
    shift-right: [w777] -> _
    shift-left: _ -> [w787]
    stop <- w778 stop-if-true
    # "TEC Peltier Controller Functions"
    n464 = Dequeue Element(queue=w776, timeout in ms (-1)="TEC monitor\nperiod (ms)") -> (element=w790:cluster{"Message":T4, "TEC ID":i32, "Data":dbl}, timed out?=w791:bool)  [unwired: 1 in, 2 out]
    n465 = case shown="True" w791 {
      tunnel: w790 -> [w809 _]
      tunnel: [w806 _] -> w778
      tunnel: [w805 w998] -> w789
      tunnel: w788 -> [w804 w998]
      tunnel: [w803 w976] -> w777
      tunnel: w787 -> [w802 w977]
      frame False {
        n466 = Unbundle By Name(w809) -> ("Message"=w808:T4, "TEC ID"=w807:i32, "Data"=w801:dbl)
        n467 = case shown="\"Auto Detect\", Default" w808 {
          tunnel: w807 -> [_ w863 w899 _ w925 w946 w964]
          tunnel: [_ _ _ TRUE _ _ _] -> w806
          tunnel: [w824 w865 w901 w918 w924 w945 w963] -> w805
          tunnel: w804 -> [w825 _ w902 w918 w924 w945 w963]
          tunnel: [w821 w862 w898 w917 w920 w939 w959] -> w803
          tunnel: w802 -> [_ w861 w897 w917 w921 w940 w960]
          tunnel: w801 -> [_ _ _ _ w926 w944 _]
          frame "Auto Detect", Default {
            w810 = FALSE
            n468 = property on="COM Done" class="Bool (strict)"("Value"=w810) -> (error out=w813:errorcluster)  [unwired: 2 in, 1 out]
            n469 = property on="TEC Done" class="Bool (strict)"(error in=w813, "Value"=w810) -> (error out=w812:errorcluster)  [unwired: 1 in, 1 out]
            n470 = property on="Auto Done" class="Bool (strict)"(error in=w812, "Value"=w810) -> (error out=w811:errorcluster)  [unwired: 1 in, 1 out]
            n471 = call "meTEC_Determine List of COM Ports.vi"("error in (no error)"=w811) -> ("error out"=w820:errorcluster, "VISA Resources List (COM Ports)"=w822:string[])  [unwired: 9 in]
            n472 = Unbundle(w820) -> ("status"=w819:bool)  [unwired: 2 out]
            n473 = call "meTEC_Find TECs.vi"("error in (no error)"=w820, "VISA Resources List (COM Ports)"=w822) -> ("error out"=w816:errorcluster, "VISA Resources List (meTEC(s))"=w823:string[])  [unwired: 8 in]
            n474 = Not(x=w819) -> (.not. x?=→"COM Done":bool)
            n475 = for {
              tunnel: w823 -> [w841] mode=indexing
              tunnel: w825 -> [w840] mode=indexing
              shift-right: [w838] -> w824
              shift-left: w825 -> [w839]
              tunnel: [w829] -> w821 mode=indexing
              tunnel: w816 -> [w837]
              tunnel: [TRUE ("Auto Done")] -> w814
              i -> [w836]
              n476 = Type Cast(type=w840, x=w841) -> (*(type *) &x=w835:refnum<visa-resource-name>)
              n477 = for {
                N: 8 -> [_]
                tunnel: [w857] -> w833 mode=indexing
                tunnel: w835 -> [w856]
                tunnel: w837 -> [w855]
                tunnel: [w851] -> w832 mode=indexing
                i -> [w854]
                n478 = Increment(x=w854) -> (x+1=w853:i32)
                n479 = Bundle("LED Controller COM Port"=w856, w853) -> (w858:T7)  [unwired: 1 in]
                n480 = call "meTEC_Read_ID 2051_Device Address.vi"("error in (no error)"=w855, "TEC Configuration_IN"=w858) -> ("error out"=w852:errorcluster, "Device Address (ID 2051) [I32]"=w857:i32)  [unwired: 7 in, 1 out]
                n481 = Unbundle(w852) -> ("status"=w851:bool)  [unwired: 2 out]
              }
              n482 = Search 1D Array(1D array=w832, element=FALSE) -> (index of element=w831:i32)  [unwired: 1 in]
              n483 = Greater Than 0?(x=w831) -> (x > 0?=w830:bool)
              n484 = case shown="False" w830 {
                tunnel: w839 -> [w842 w850]
                tunnel: [w842 w849] -> w838
                tunnel: w835 -> [_ w848]
                tunnel: w833 -> [_ w847]
                tunnel: w831 -> [_ w845]
                tunnel: [FALSE TRUE] -> w829
                frame False {
                }
                frame True {
                  n485 = Index Array(array=w847, index=w845) -> (element=w846:i32)
                  n486 = Replace Array Subset(array=w850, new element=w848, index=w846) -> (w849:refnum<visa-resource-name>[])
                }
              }
              "index" <- w836
            }
            "Auto Done" <- w814
            n487 = Unbundle(w816) -> ("status"=w817:bool)  [unwired: 2 out]
            n488 = Not(x=w817) -> (.not. x?=→"TEC Done":bool)
            n489 = for {
              tunnel: w822 -> [w826] mode=indexing
              tunnel: w821 -> [_] mode=indexing
              n490 = VISA Unlock(11:w826) -> ()  [unwired: 1 in, 2 out]
            }
            n491 = property on="TEC COM Ports" class="Arr (strict)"("Value"=w824) -> ()  [unwired: 2 in, 2 out]
          }
          frame "Connect" {
            n492 = Decrement(x=w863) -> (x-1=w860:i32)
            n493 = Not Equal To 0?(x=w863) -> (x != 0?=w864:bool)
            n494 = case shown="True" w864 {
              tunnel: w860 -> [_ w883]
              tunnel: "TEC COM Ports" -> [w868 w880]
              tunnel: [w867 w879] -> w865
              tunnel: [w866 w875] -> w862
              tunnel: w861 -> [_ w876]
              frame False {
                n495 = for {
                  tunnel: w868 -> [w871] mode=indexing
                  tunnel: [w873] -> w867 mode=indexing
                  tunnel: [w869] -> w866 mode=indexing
                  n496 = call "meTEC_Open Session.vi"("COM Port"=w871) -> ("error out"=w874:errorcluster, "VISA resource name_OUT"=w872:refnum<visa-resource-name>)  [unwired: 9 in]
                  n497 = Unbundle By Name(w874) -> ("status"=w870:bool)
                  n498 = Select(t=w871, s=w870, f=w872) -> (s? t:f=w873:refnum<visa-resource-name>)
                  n499 = Not(x=w870) -> (.not. x?=w869:bool)
                }
              }
              frame True {
                n500 = To Long Integer(number=w883) -> (32bit integer=w878:i32)
                n501 = Index Array(array=w880, index=w878) -> (element=w882:refnum<visa-resource-name>)
                n502 = call "meTEC_Open Session.vi"("COM Port"=w882) -> ("error out"=w877:errorcluster, "VISA resource name_OUT"=w881:refnum<visa-resource-name>)  [unwired: 9 in]
                n503 = case shown="No Error" w877 {
                  tunnel: w881 -> [w890 _]
                  tunnel: w880 -> [w889 w895]
                  tunnel: [w888 w895] -> w879
                  tunnel: w878 -> [w887 w892]
                  tunnel: w876 -> [w886 w894]
                  tunnel: [w885 w893] -> w875
                  frame No Error {
                    n504 = Replace Array Subset(array=w889, new element=w890, index=w887) -> (w888:refnum<visa-resource-name>[])
                    n505 = Replace Array Subset(array=w886, new element=TRUE ("new element/subarray"), index=w887) -> (w885:bool[])
                  }
                  frame Error {
                    n506 = Replace Array Subset(array=w894, new element=FALSE ("new element/subarray"), index=w892) -> (w893:bool[])
                  }
                }
              }
            }
          }
          frame "Disconnect" {
            n507 = Decrement(x=w899) -> (x-1=w896:i32)
            n508 = Not Equal To 0?(x=w899) -> (x != 0?=w900:bool)
            n509 = case shown="True" w900 {
              tunnel: w896 -> [_ w916]
              tunnel: w902 -> [w905 w910]
              tunnel: [w904 w910] -> w901
              tunnel: [w903 w914] -> w898
              tunnel: w897 -> [_ w915]
              frame False {
                n510 = for {
                  tunnel: w905 -> [w908] mode=indexing
                  tunnel: [w908] -> w904 mode=indexing
                  tunnel: [FALSE] -> w903 mode=indexing
                  n511 = VISA Close(VISA resource name=w908) -> (error out=w906:errorcluster)  [unwired: 1 in]
                  n512 = call <vilib>:"Clear Errors.vi"("error in (no error)"=w906) -> ()  [unwired: 5 in, 2 out]
                }
              }
              frame True {
                n513 = To Long Integer(number=w916) -> (32bit integer=w909:i32)
                n514 = Index Array(array=w910, index=w909) -> (element=w913:refnum<visa-resource-name>)
                n515 = VISA Close(VISA resource name=w913) -> (error out=w911:errorcluster)  [unwired: 1 in]
                n516 = call <vilib>:"Clear Errors.vi"("error in (no error)"=w911) -> ()  [unwired: 5 in, 2 out]
                n517 = Replace Array Subset(array=w915, new element=FALSE ("new element/subarray"), index=w909) -> (w914:bool[])
              }
            }
          }
          frame "Exit" {
          }
          frame "Set Temp" {
            n518 = Decrement(x=w925) -> (x-1=w923:i32)
            n519 = Index Array(array=w921, index=w923) -> (element=w922:bool)
            n520 = case shown="True" w922 {
              tunnel: w926 -> [_ w936]
              tunnel: w925 -> [_ w935]
              tunnel: w924 -> [_ w934]
              tunnel: w923 -> [_ w932]
              tunnel: w921 -> [w927 w931]
              tunnel: [w927 w930] -> w920
              frame False {
              }
              frame True {
                n521 = Index Array(array=w934, index=w932) -> (element=w938:refnum<visa-resource-name>)
                n522 = Bundle("LED Controller COM Port"=w938, "TEC ID"=w935) -> (w937:T8)  [unwired: 1 in]
                n523 = call "meTEC_Set_ID 3000_Object Target Temperature.vi"("TEC Configuration_IN"=w937, "Object Target Temperature [°C]"=w936) -> ("error out"=w933:errorcluster)  [unwired: 7 in, 2 out]
                n524 = Unbundle(w933) -> ("status"=w929:bool)  [unwired: 2 out]
                n525 = Not(x=w929) -> (.not. x?=w928:bool)
                n526 = Replace Array Subset(array=w931, new element=w928, index=w932) -> (w930:bool[])
              }
            }
          }
          frame "Output Ena" {
            n527 = Decrement(x=w946) -> (x-1=w942:i32)
            n528 = Index Array(array=w940, index=w942) -> (element=w941:bool)
            n529 = To Long Integer(number=w944) -> (32bit integer=w943:i32)
            n530 = case shown="True" w941 {
              tunnel: w946 -> [_ w957]
              tunnel: w942 -> [_ w950]
              tunnel: w945 -> [_ w956]
              tunnel: w943 -> [_ w954]
              tunnel: w940 -> [w947 w952]
              tunnel: [w947 w951] -> w939
              frame False {
              }
              frame True {
                n531 = Index Array(array=w956, index=w950) -> (element=w958:refnum<visa-resource-name>)
                n532 = Bundle("LED Controller COM Port"=w958, "TEC ID"=w957) -> (w955:T8)  [unwired: 1 in]
                n533 = call "meTEC_Set_ID 50000_Live Enable.vi"("TEC Configuration_IN"=w955, "Live Enable (ID 50000)"=w954) -> ("error out"=w953:errorcluster)  [unwired: 7 in, 2 out]
                n534 = Unbundle(w953) -> ("status"=w949:bool)  [unwired: 2 out]
                n535 = Not(x=w949) -> (.not. x?=w948:bool)
                n536 = Replace Array Subset(array=w952, new element=w948, index=w950) -> (w951:bool[])
              }
            }
          }
          frame "RESET" {
            n537 = Decrement(x=w964) -> (x-1=w962:i32)
            n538 = Index Array(array=w960, index=w962) -> (element=w961:bool)
            n539 = case shown="True" w961 {
              tunnel: w964 -> [_ w974]
              tunnel: w962 -> [_ w966]
              tunnel: w963 -> [_ w973]
              tunnel: w960 -> [w965 w971]
              tunnel: [w965 w970] -> w959
              frame False {
              }
              frame True {
                n540 = Index Array(array=w973, index=w966) -> (element=w975:refnum<visa-resource-name>)
                n541 = Bundle("LED Controller COM Port"=w975, "TEC ID"=w974) -> (w972:T8)  [unwired: 1 in]
                n542 = call "meTEC_Reset Device.vi"("TEC Configuration_IN"=w972) -> ("error out"=w969:errorcluster)  [unwired: 8 in, 2 out]
                n543 = Unbundle(w969) -> ("status"=w968:bool)  [unwired: 2 out]
                n544 = Not(x=w968) -> (.not. x?=w967:bool)
                n545 = Replace Array Subset(array=w971, new element=w967, index=w966) -> (w970:bool[])
              }
            }
          }
        }
      }
      frame True {
        n546 = for {
          tunnel: w998 -> [w1006] mode=indexing
          tunnel: [w1003] -> w981 mode=indexing
          tunnel: w977 -> [w1002] mode=indexing
          tunnel: [w1001] -> w983 mode=indexing
          tunnel: [w1000] -> w982 mode=indexing
          tunnel: [w999] -> w978 mode=indexing
          i -> [w1005]
          n547 = Increment(x=w1005) -> (x+1=w1004:i32)
          n548 = case shown="True" w1002 {
            tunnel: w1006 -> [_ w1018]
            tunnel: w1004 -> [_ w1011]
            tunnel: [w1008 w1017] -> w1003
            tunnel: [w1008 w1013] -> w1001
            tunnel: [w1008 w1012] -> w1000
            tunnel: [TRUE ("status") w1009] -> w999
            frame False {
              w1008 = nan ("Object Temperature [°C] (ID 1000)")
            }
            frame True {
              n549 = Bundle("LED Controller COM Port"=w1018, w1011) -> (w1016:T7)  [unwired: 1 in]
              n550 = call "meTEC_Read_ID 1000_Object Temperature.vi"("TEC Configuration_IN"=w1016) -> ("error out"=w1015:errorcluster, "Object Temperature [°C] (ID 1000)"=w1017:dbl)  [unwired: 8 in, 1 out]
              n551 = call "meTEC_Read_ID 1020_Actual Output Current.vi"("error in (no error)"=w1015, "TEC Configuration_IN"=w1016) -> ("error out"=w1014:errorcluster, "Act. Output Current [A] (ID 1020)"=w1013:dbl)  [unwired: 7 in, 1 out]
              n552 = call "meTEC_Read_ID 1021_Actual Output Voltage.vi"("error in (no error)"=w1014, "TEC Configuration_IN"=w1016) -> ("error out"=w1010:errorcluster, "Act. Output Voltage [A] (ID 1021)"=w1012:dbl)  [unwired: 7 in, 1 out]
              n553 = Unbundle(w1010) -> ("status"=w1009:bool)  [unwired: 2 out]
            }
          }
        }
        "TEC Current" <- w983
        "TEC Voltage" <- w982
        "TempArray" <- w981
        n554 = Not(x=w978) -> (.not. x?=w976:bool[])
        n555 = Index Array(array=w981) -> (element #1=→"cell 1A actual":dbl, element #2=→"cell 2A actual":dbl, element #3=→"cell 3A actual":dbl, element #4=→"cell 4A actual":dbl, element #5=→"cell 1B actual":dbl, element #6=→"cell 2B actual":dbl, element #7=→"cell 3B actual":dbl, element #8=→"cell 4B actual":dbl)  [unwired: 8 in]
        n556 = Array Subset(array=w981, index=4, length=4) -> (w984:dbl[])
        n557 = Array Subset(array=w981, index=0, length=4) -> (w987:dbl[])
        n558 = Build Array(w984) -> (→"Temperature Monitor B":dbl[][])
        n559 = Build Array(w987) -> (→"Temperature Monitor A":dbl[][])
      }
    }
    "TEC COM Status" <- w777
    n560 = Index Array(array=w777) -> (element #1=→"TEC 1A Status":bool, element #2=→"TEC 2A Status":bool, element #3=→"TEC 3A Status":bool, element #4=→"TEC 4A Status":bool, element #5=→"TEC 1B Status":bool, element #6=→"TEC 2B Status":bool, element #7=→"TEC 3B Status":bool, element #8=→"TEC 4B Status":bool)  [unwired: 8 in]
    n561 = for {
      tunnel: w777 -> [w795] mode=indexing
      tunnel: w776 -> [w796]
      tunnel: "TEC Auto-Connect" -> [w793]
      i -> [w798]
      n562 = Increment(x=w798) -> (x+1=w797:i32)
      n563 = Compound Arithmetic op=AND(w793, invert w795) -> (w794:bool)
      n564 = case shown="True" w794 {
        tunnel: w797 -> [_ w800]
        tunnel: w796 -> [_ w799]
        frame False {
        }
        frame True {
          n565 = call "TEC COM Reconnect.vi"("TEC ID"=w800, "queue in"=w799) -> ()  [unwired: 9 in, 1 out]
        }
      }
    }
  }
  n566 = while {
    stop <- w1019 stop-if-true
    n567 = event shown="[7] \"TimingList1\": Edit Cell" {
      selector: _ -> [_ _ _ _ _ _ _ _]
      dyn-events: _ -> [_ _ _ _ _ _ _ _]
      timeout: _ -> [_ _ _ _ _ _ _ _]
      tunnel: [_ _ _ _ TRUE _ _ _] -> w1019
      event "LoadControlTable": Value Change {
        n568 = event-data() -> ()  [unwired: 1 in, 5 out]
        n569 = call-poly <vilib>:"Read Delimited Spreadsheet.vi"("delimiter (\\t)"="," ("delimiter (\\t)")) -> ("all rows"=w1022:string[][])  [unwired: 9 in, 5 out]
        n570 = property on="TimingList1" class="MCListbox (strict)"("ItemNames"=w1022) -> ()  [unwired: 2 in, 2 out]
        n571 = Fract/Exp String To Number(string=w1022) -> (number=w1021:dbl[][])  [unwired: 3 in, 1 out]
        n572 = local write "ControlTable1"(w1021) -> ()
      }
      event "SaveControlTable": Value Change {
        n573 = event-data() -> ()  [unwired: 1 in, 6 out]
        n574 = local read "ControlTable1"() -> (w1024:dbl[][])
        n575 = call-poly <vilib>:"Write Delimited Spreadsheet.vi"("2D data"=w1024, "delimiter (\\t)"="," ("delimiter (\\t)")) -> ()  [unwired: 12 in, 2 out]
      }
      event "AddRow1": Value Change {
        n576 = event-data() -> ()  [unwired: 1 in, 6 out]
        n577 = property on="TimingList1" class="MCListbox (strict)"() -> ("ItemNames"=w1031:string[][], "Value"=w1026:i32)  [unwired: 2 in, 2 out]
        n578 = Greater Or Equal?(x=w1026, y=0) -> (x >= y?=w1028:bool)
        n579 = case shown="False" w1028 {
          tunnel: w1031 -> [_ w1038]
          tunnel: w1026 -> [_ w1037]
          tunnel: [string[] ["0", "0", "20", "20", "20", "20", "00000000", "00000000", "00000000"] ("Item Names") w1036] -> w1030
          tunnel: w1026 -> [_ w1035]
          tunnel: [0 ("Value") w1035] -> w1025
          frame False {
          }
          frame True {
            n580 = Index Array(array=w1038, index (row)=w1037) -> (element=w1036:string[])  [unwired: 1 in]
          }
        }
        n581 = Insert Into Array(array=w1031, index (row)=w1025, new element=w1030) -> (w1029:string[][])  [unwired: 1 in]
        n582 = Fract/Exp String To Number(string=w1029) -> (number=w1032:dbl[][])  [unwired: 3 in, 1 out]
        n583 = local write "ControlTable1"(w1032) -> ()
        n584 = property on="TimingList1" class="MCListbox (strict)"("ItemNames"=w1029) -> ()  [unwired: 2 in, 2 out]
      }
      event "RemoveRow1": Value Change {
        n585 = event-data() -> ()  [unwired: 1 in, 6 out]
        n586 = property on="TimingList1" class="MCListbox (strict)"() -> ("ItemNames"=w1041:string[][], "Value"=w1040:i32)  [unwired: 2 in, 2 out]
        n587 = Delete From Array(array=w1041, index (row)=w1040) -> (array with subset deleted=w1039:string[][])  [unwired: 2 in, 1 out]
        n588 = Fract/Exp String To Number(string=w1039) -> (number=w1042:dbl[][])  [unwired: 3 in, 1 out]
        n589 = local write "ControlTable1"(w1042) -> ()
        n590 = property on="TimingList1" class="MCListbox (strict)"("ItemNames"=w1039) -> ()  [unwired: 2 in, 2 out]
      }
      event "stop": Value Change {
        n591 = event-data() -> ()  [unwired: 1 in, 6 out]
      }
      event "StartMagicControl": Value Change {
        n592 = event-data() -> ()  [unwired: 1 in, 6 out]
        n593 = Get Date/Time In Seconds() -> (seconds since 1Jan1904=w1044:timestamp)
        "started at" <- w1044
        n594 = property on="StopMagicControl" class="Bool"("DisabledEnum"=T6."Enabled" ("Disabled")) -> ()  [unwired: 2 in, 2 out]
        n595 = property on="StartMagicControl" class="Bool"("DisabledEnum"=T6."Disabled and Grayed Out" ("Disabled")) -> ()  [unwired: 2 in, 2 out]
        n596 = local write "started last"(w1044) -> ()
        "Automatic Control Active H1" <- TRUE ("Automatic Control Active")
        "Active Row" <- -1
      }
      event "StopMagicControl": Value Change {
        n597 = event-data() -> ()  [unwired: 1 in, 6 out]
        n598 = local write "Automatic Control Active H1"(FALSE ("Automatic Control Active")) -> ()
        n599 = property on="StartMagicControl" class="Bool"("DisabledEnum"=T6."Enabled" ("Disabled")) -> ()  [unwired: 2 in, 2 out]
        n600 = property on="StopMagicControl" class="Bool"("DisabledEnum"=T6."Disabled and Grayed Out" ("Disabled")) -> ()  [unwired: 2 in, 2 out]
      }
      event "TimingList1": Edit Cell {
        n601 = event-data() -> ()  [unwired: 1 in, 6 out]
        n602 = property on="TimingList1" class="MCListbox (strict)"() -> ("ItemNames"=w1053:string[][])  [unwired: 2 in, 2 out]
        n603 = Fract/Exp String To Number(string=w1053) -> (number=→"ControlTable1":dbl[][])  [unwired: 3 in, 1 out]
      }
    }
    "stopped" <- w1019
  }
  n604 = while {
    stop <- w1054 stop-if-true
    n605 = event shown="[1] \"SaveControlTable 2\": Value Change" {
      selector: _ -> [_ _ _ _ _ _ _ _]
      dyn-events: _ -> [_ _ _ _ _ _ _ _]
      timeout: _ -> [_ _ _ _ _ _ _ _]
      tunnel: [_ _ _ _ TRUE _ _ _] -> w1054
      event "LoadControlTable 2": Value Change {
        n606 = event-data() -> ()  [unwired: 1 in, 5 out]
        n607 = call-poly <vilib>:"Read Delimited Spreadsheet.vi"("delimiter (\\t)"="," ("delimiter (\\t)")) -> ("all rows"=w1056:string[][])  [unwired: 9 in, 5 out]
        n608 = property on="TimingList2" class="MCListbox (strict)"("ItemNames"=w1056) -> ()  [unwired: 2 in, 2 out]
        n609 = Fract/Exp String To Number(string=w1056) -> (number=w1057:dbl[][])  [unwired: 3 in, 1 out]
        n610 = local write "ControlTable2"(w1057) -> ()
      }
      event "SaveControlTable 2": Value Change {
        n611 = event-data() -> ()  [unwired: 1 in, 6 out]
        n612 = local read "ControlTable2"() -> (w1059:dbl[][])
        n613 = call-poly <vilib>:"Write Delimited Spreadsheet.vi"("2D data"=w1059, "delimiter (\\t)"="," ("delimiter (\\t)")) -> ()  [unwired: 12 in, 2 out]
      }
      event "AddRow2": Value Change {
        n614 = event-data() -> ()  [unwired: 1 in, 6 out]
        n615 = property on="TimingList2" class="MCListbox (strict)"() -> ("ItemNames"=w1060:string[][], "Value"=w1061:i32)  [unwired: 2 in, 2 out]
        n616 = Greater Or Equal?(x=w1061, y=0) -> (x >= y?=w1065:bool)
        n617 = case shown="False" w1065 {
          tunnel: w1060 -> [_ w1073]
          tunnel: w1061 -> [_ w1072]
          tunnel: [string[] ["0", "0", "20", "20", "20", "20", "00000000", "00000000", "00000000"] ("Item Names") w1071] -> w1066
          tunnel: w1061 -> [_ w1070]
          tunnel: [0 ("Value") w1070] -> w1063
          frame False {
          }
          frame True {
            n618 = Index Array(array=w1073, index (row)=w1072) -> (element=w1071:string[])  [unwired: 1 in]
          }
        }
        n619 = Insert Into Array(array=w1060, index (row)=w1063, new element=w1066) -> (w1062:string[][])  [unwired: 1 in]
        n620 = Fract/Exp String To Number(string=w1062) -> (number=w1067:dbl[][])  [unwired: 3 in, 1 out]
        n621 = local write "ControlTable2"(w1067) -> ()
        n622 = property on="TimingList2" class="MCListbox (strict)"("ItemNames"=w1062) -> ()  [unwired: 2 in, 2 out]
      }
      event "RemoveRow2": Value Change {
        n623 = event-data() -> ()  [unwired: 1 in, 6 out]
        n624 = property on="TimingList2" class="MCListbox (strict)"() -> ("ItemNames"=w1076:string[][], "Value"=w1075:i32)  [unwired: 2 in, 2 out]
        n625 = Delete From Array(array=w1076, index (row)=w1075) -> (array with subset deleted=w1074:string[][])  [unwired: 2 in, 1 out]
        n626 = Fract/Exp String To Number(string=w1074) -> (number=w1077:dbl[][])  [unwired: 3 in, 1 out]
        n627 = local write "ControlTable2"(w1077) -> ()
        n628 = property on="TimingList2" class="MCListbox (strict)"("ItemNames"=w1074) -> ()  [unwired: 2 in, 2 out]
      }
      event "stop": Value Change {
        n629 = event-data() -> ()  [unwired: 1 in, 6 out]
      }
      event "StartMagicControl 2": Value Change {
        n630 = event-data() -> ()  [unwired: 1 in, 6 out]
        n631 = Get Date/Time In Seconds() -> (seconds since 1Jan1904=w1081:timestamp)
        "started at 2" <- w1081
        n632 = property on="StopMagicControl 2" class="Bool"("DisabledEnum"=T6."Enabled" ("Disabled")) -> ()  [unwired: 2 in, 2 out]
        n633 = property on="StartMagicControl 2" class="Bool"("DisabledEnum"=T6."Disabled and Grayed Out" ("Disabled")) -> ()  [unwired: 2 in, 2 out]
        n634 = local write "started last 2"(w1081) -> ()
        "Active Row 2" <- -1
        "Automatic Control Active H2" <- TRUE ("Automatic Control Active")
      }
      event "StopMagicControl 2": Value Change {
        n635 = event-data() -> ()  [unwired: 1 in, 6 out]
        n636 = local write "Automatic Control Active H2"(FALSE ("Automatic Control Active")) -> ()
        n637 = property on="StartMagicControl 2" class="Bool"("DisabledEnum"=T6."Enabled" ("Disabled")) -> ()  [unwired: 2 in, 2 out]
        n638 = property on="StopMagicControl 2" class="Bool"("DisabledEnum"=T6."Disabled and Grayed Out" ("Disabled")) -> ()  [unwired: 2 in, 2 out]
      }
      event "TimingList2": Edit Cell {
        n639 = event-data() -> ()  [unwired: 1 in, 6 out]
        n640 = property on="TimingList2" class="MCListbox (strict)"() -> ("ItemNames"=w1087:string[][])  [unwired: 2 in, 2 out]
        n641 = Fract/Exp String To Number(string=w1087) -> (number=→"ControlTable2":dbl[][])  [unwired: 3 in, 1 out]
      }
    }
  }
